vi "main_ui.vi"() -> ()   [LabVIEW 2018]
uses:
  <vilib>/Utility/miscctls.llb/LVPointDoubleTypeDef.ctl
  <vilib>/Analysis/1siggen.llb/Ramp Pattern by Samples.vi
  src/GLOBAL_VAR.vi
  <vilib>/Analysis/NI_AALBase.lvlib
panel:
  in  "T2_open":bool caption="Open T1"
  in  "parameters_z-scan":T1={"dwell_time_ms"=10.0, "q_steps"=20, "span_um"=2.0, "refocus"=TRUE}
  in  "parameters_xy-scan":T2={"image_size_xy_um"=0.5, "frame_size_xy_px"=20, "dwell_time_ms"=1.0}
  in  "continious_recenter":bool
  in  "recenter":bool caption="Laser"
  out "Laser power [mW]":dbl caption="Power" format="%.3f"
  in  "laser_on-off":bool caption="Laser"
  in  "T1_open":bool caption="Open T1"
  in  "esr_start":bool caption="Open ESR"
  in  "stop":bool
  in  "scan_start":bool
  in  "live-scan":bool
  out "ESR_stack":dbl[][](graph)
  out "X":dbl caption="X Rel" format="%.3f"
  out "Y":dbl caption="Y Rel" format="%.3f"
  out "XY Graph 2":cluster{"Value":dbl[], "Ramp Pattern":dbl[]}(graph)={"Value"=[-75.0, -71.93877551020408, -68.87755102040816, -65.81632653061224, -62.755102040816325, -59.69387755102041, -56.63265306122449, -53.57142857142857, -50.51020408163265, -47.44897959183673, -44.38775510204081, -41.3265306122449, -38.26530612244898, -35.204081632653065, -32.142857142857146, -29.081632653061227, -26.02040816326531, -22.95918367346939, -19.89795918367347, -16.836734693877553, -13.775510204081634, -10.714285714285722, -7.653061224489804, -4.591836734693885, -1.5306122448979664, 1.5306122448979522, 4.591836734693871, 7.6530612244897895, 10.714285714285708, 13.775510204081627, 16.836734693877546, 19.897959183673464, 22.959183673469383, 26.0204081632653, 29.08163265306122, 32.14285714285714, 35.20408163265306, 38.265306122448976, 41.326530612244895, 44.38775510204081, 47.44897959183673, 50.51020408163265, 53.571428571428555, 56.63265306122449, 59.69387755102039, 62.755102040816325, 65.81632653061223, 68.87755102040816, 71.93877551020407, 75.0], "Ramp Pattern"=[0.0, 0.0, 0.0, 0.0, 0.0, 0.0, 0.0, 0.0, 0.0, 0.0, 0.0, 0.0, 0.0, 0.0, 0.0, 0.0, 0.0, 0.0, 0.0, 0.0, 0.0, 0.0, 0.0, 0.0, 0.0, 0.0, 0.0, 0.0, 0.0, 0.0, 0.0, 0.0, 0.0, 0.0, 0.0, 0.0, 0.0, 0.0, 0.0, 0.0, 0.0, 0.0, 0.0, 0.0, 0.0, 0.0, 0.0, 0.0, 0.0, 0.0]}
  out "XY Graph":cluster{"Value":dbl[], "Ramp Pattern":dbl[]}(graph)={"Value"=[0.0, 0.0, 0.0, 0.0, 0.0, 0.0, 0.0, 0.0, 0.0, 0.0, 0.0, 0.0, 0.0, 0.0, 0.0, 0.0, 0.0, 0.0, 0.0, 0.0, 0.0, 0.0, 0.0, 0.0, 0.0, 0.0, 0.0, 0.0, 0.0, 0.0, 0.0, 0.0, 0.0, 0.0, 0.0, 0.0, 0.0, 0.0, 0.0, 0.0, 0.0, 0.0, 0.0, 0.0, 0.0, 0.0, 0.0, 0.0, 0.0, 0.0], "Ramp Pattern"=[-75.0, -71.93877551020408, -68.87755102040816, -65.81632653061224, -62.755102040816325, -59.69387755102041, -56.63265306122449, -53.57142857142857, -50.51020408163265, -47.44897959183673, -44.38775510204081, -41.3265306122449, -38.26530612244898, -35.204081632653065, -32.142857142857146, -29.081632653061227, -26.02040816326531, -22.95918367346939, -19.89795918367347, -16.836734693877553, -13.775510204081634, -10.714285714285722, -7.653061224489804, -4.591836734693885, -1.5306122448979664, 1.5306122448979522, 4.591836734693871, 7.6530612244897895, 10.714285714285708, 13.775510204081627, 16.836734693877546, 19.897959183673464, 22.959183673469383, 26.0204081632653, 29.08163265306122, 32.14285714285714, 35.20408163265306, 38.265306122448976, 41.326530612244895, 44.38775510204081, 47.44897959183673, 50.51020408163265, 53.571428571428555, 56.63265306122449, 59.69387755102039, 62.755102040816325, 65.81632653061223, 68.87755102040816, 71.93877551020407, 75.0]}
  out "scan_image":dbl[][](graph)
  out "wavechart_01":dbl(graph)
  in  "Tab Control":T3(tab)
  in  "counting_start":bool
  out "counts":dbl format="%.3e"
  in  "counts_dwell_time":dbl=30.0 caption="Dwell time [ms] :" min=0.0
  in  "pos-zero":bool caption="Blank Button"
  in  "scan_direction":enum32{"0", "1"}(radio)=enum."1" caption="Scan direction:"
  in  "frame_size_x_px":i32=100 caption="image_size_x"
  out "frame_size_y_px":i32=100 caption="image_size_y"
  out "pixel_size_z_um":dbl format="%#_3g"
  out "pixel_size_x_um":dbl=1.5 format="%#_3g"
  out "pixel_size_y_um":dbl=1.5 format="%#_3g"
  in  "pixel_dwell_ms":dbl=1.0 caption="Dwell time:"
  out "time_frame_s":dbl=10.0 caption="Time per frame:"
  in  "cursor-reset":bool caption="Blank Button"
  in  "pos-start_y":dbl caption="Y:" format="%#.3g"
  in  "pos-start_x":dbl caption="X:" format="%#.3f"
  in  "pos-start_cursor":bool caption="Blank Button"
  in  "pos_start":enum32{"bottom-left", "center"}(radio)=enum."center"
  in  "image_size_x_um":dbl=150.0 caption="X:"
  out "image_size_y_um":dbl=150.0 caption="Y:"
  in  "pos_z":dbl(slide) caption="Z:" scale=0.0..200.0
  in  "focus_z":dbl caption="Focus :" min=0.0 max=200.0 step=0.001 format="%.3f"
  in  "focus_dwell_ms":dbl=100.0 caption="Dwell :"
  in  "focus_q_steps":i32=100 caption="Steps :"
  in  "focus_z_end":dbl=100.0 caption="End :"
  in  "focus_z_start":dbl caption="Start :"
  in  "focus_start":bool
  out "timeseries-rem_time":string caption="Remaining time :"
  in  "timeseries-autofocus":enum16{"No autofocus", "Max x-y", "Center"}(ring) caption="Autofocus :"
  out "timeseries-current_image":dbl caption="Current scan :" format="%#.3f"
  out "timeseries-total_images":dbl=1.0 caption="Total scans :" format="%#.3f"
  in  "timeseries-start":bool
  in  "timeseries-period":dbl caption="Period :" format="%#.3f"
  in  "timeseries-stopdate":timestamp=timestamp(3557915984.536238 s since 1904-01-01) caption="Stop at :" format="%<%X\n%x>T"
  out "timeseries-next_scan":timestamp caption="Next scan at :" format="%<%X\n%x>T"
  in  "Z-stack_enable":bool
  in  "z-stack_slices":i32=1 caption="Slices :" min=1 step=1
  out "z-stack_step_size":dbl caption="Step size :" format="%#.4f"
  in  "Z-stack_tabs":enum32{"From-To", "Centering"}(tab)
  in  "z-stack-set_to":bool
  in  "z-stack-set_from":bool
  in  "z-stack_to":dbl=100.0 caption="To :"
  in  "z-stack_from":dbl caption="From :"
  in  "z-stack-set_center":bool
  in  "z-stack_size":dbl=10.0 caption="Size :"
  in  "z-stack_center":dbl=5.0 caption="Center :"
  in  "z-stack_pos":i32(slide)=1 caption="Z slice :" min=1 step=1 scale=1.0..1.1
  in  "current_z":dbl caption="Z :" min=0.0 max=100.0 step=0.0001 format="%.4f"
  in  "current_y":dbl caption="Y :" min=-10.0 max=10.0 step=0.0001 format="%.4f"
  in  "current_x":dbl caption="X :" min=-10.0 max=10.0 step=0.0001 format="%.4f"
  in  "XY Max focus?":bool
  in  "X Zero":dbl format="%.3f"
  in  "Y Zero":dbl format="%.3f"
  in  "X Rel":dbl format="%.3f"
  in  "Y Rel":dbl format="%.3f"
  out "upos-xy_control":cluster{"X":dbl, "Y":dbl}[](graph)
  in  "upos-stop":bool
  in  "upos-x":dbl caption="X:" min=0.0 max=7.0 format="%.3f"
  in  "upos-y":dbl caption="Y:" min=0.0 max=7.0 format="%.3f"
  out "upos-cpos_y":dbl format="%#.3f"
  out "upos-cpos_x":dbl format="%#.3f"
  out "upos-state_x":u32 caption="X:"
  out "upos-state_y":u32 caption="Y:"
  in  "tiles-overlap":dbl=10.0 caption="Overlap :"
  out "tile_progress":u8(slide) caption="Progress :" scale=0.0..100.0
  out "tile_remaining_tiles":dbl caption="Remaining\ntiles :"
  out "tile_remaining_time":dbl caption="Remaining\ntime :"
  in  "tile-scan_start":bool
  in  "tile_tiles-size":enum32{"tiles", "size"}(radio)=enum."size"
  out "tile_q-tiles_y":dbl=1.0 caption="Y :"
  in  "tile_q-tiles_x":dbl=1.0 caption="X :"
  out "tile_size_y_um":dbl=10.0 caption="Y:"
  in  "tile_size_x_um":dbl=10.0 caption="Size :"
  in  "tile_start_y_mm":dbl caption="Y:" format="%#.3g"
  in  "tile_start_x_mm":dbl caption="X:" format="%#.3f"
  out "esr_generator_ok":bool caption="Generator\nstatus :"
  out "esr_current_run":i32 caption="Run :"
  in  "esr_out_enable":bool caption="Output on/off :"
  out "esr_power_led":bool
  out "esr_remain":i32 caption="Remain :"
  in  "esr_repetitions":i32=1 caption="Repetitions" min=1 max=1000 step=1
  in  "esr_dwell_time":ext=0.09999999974525053 caption="Dwell Time :" format="%.3f"
  in  "esr_step_size":ext=2500000.0 caption="Step size :" format="%.2p"
  in  "esr_freq_stop":ext=3000000000.0 caption="Freq Stop :" format="%.2p"
  in  "esr_freq_start":ext=2800000000.0 caption="Freq Start :" format="%.2p"
  out "esr_total_time":ext=8120.249980327117 caption="Total time :"
  in  "esr_power":ext=5.999999061226845 caption="Power :" format="%.2f"
  in  "live_scan_direction":enum32{"0", "1"}(radio)=enum."1" caption="Scan direction:"
  in  "live_frame_size_x_px":i32=50 caption="image_size_x"
  in  "live_pixel_dwell_ms":dbl=0.5 caption="Dwell time:"
  in  "objective":u16(ring)=1 items=["Raw scale (volts)", "UPlanSApo 100x / 1,40 Oil", "UPlanSApo 40X / 0,95 Air"]
  in  "file_save":bool
  in  "file_autosave":bool
  in  "file_path":path caption="Folder :"
  in  "file_name":string caption="Name :"
  in  "save_tiff":bool
  in  "save_txt":bool
  # "Relative cursor position [um]"
  # "Scanning area [mm]"
  # "Size:"
  # "x"
  # "Position:"
  # "Acquisition"
  # "Frame size:"
  # "x"
  # "px"
  # "ms"
  # "Pixel size [mm] :"
  # "x"
  # "x"
  # "Seconds"
  # "Manual focus [mm]"
  # "Auto-focus [mm]"
  # "ms"
  # "Photon counting"
  # "Time series"
  # "[s]"
  # "Z stack [mm]"
  # "Set position [mm]"
  # "Positioners (xy motors)"
  # "Absolute"
  # "Zeros"
  # "Relative"
  # "Status"
  # "State :"
  # "Position :"
  # "Tiles scan"
  # "Start position [mm]:"
  # "mm"
  # "mm"
  # "mm"
  # "min"
  # "Sweep"
  # "Hz"
  # "Hz"
  # "Hz"
  # "ms"
  # "dBm"
  # "s"
  # "Objective"
  # "Live scan"
  # "Frame size:"
  # "px"
  # "ms"
  # "Save"
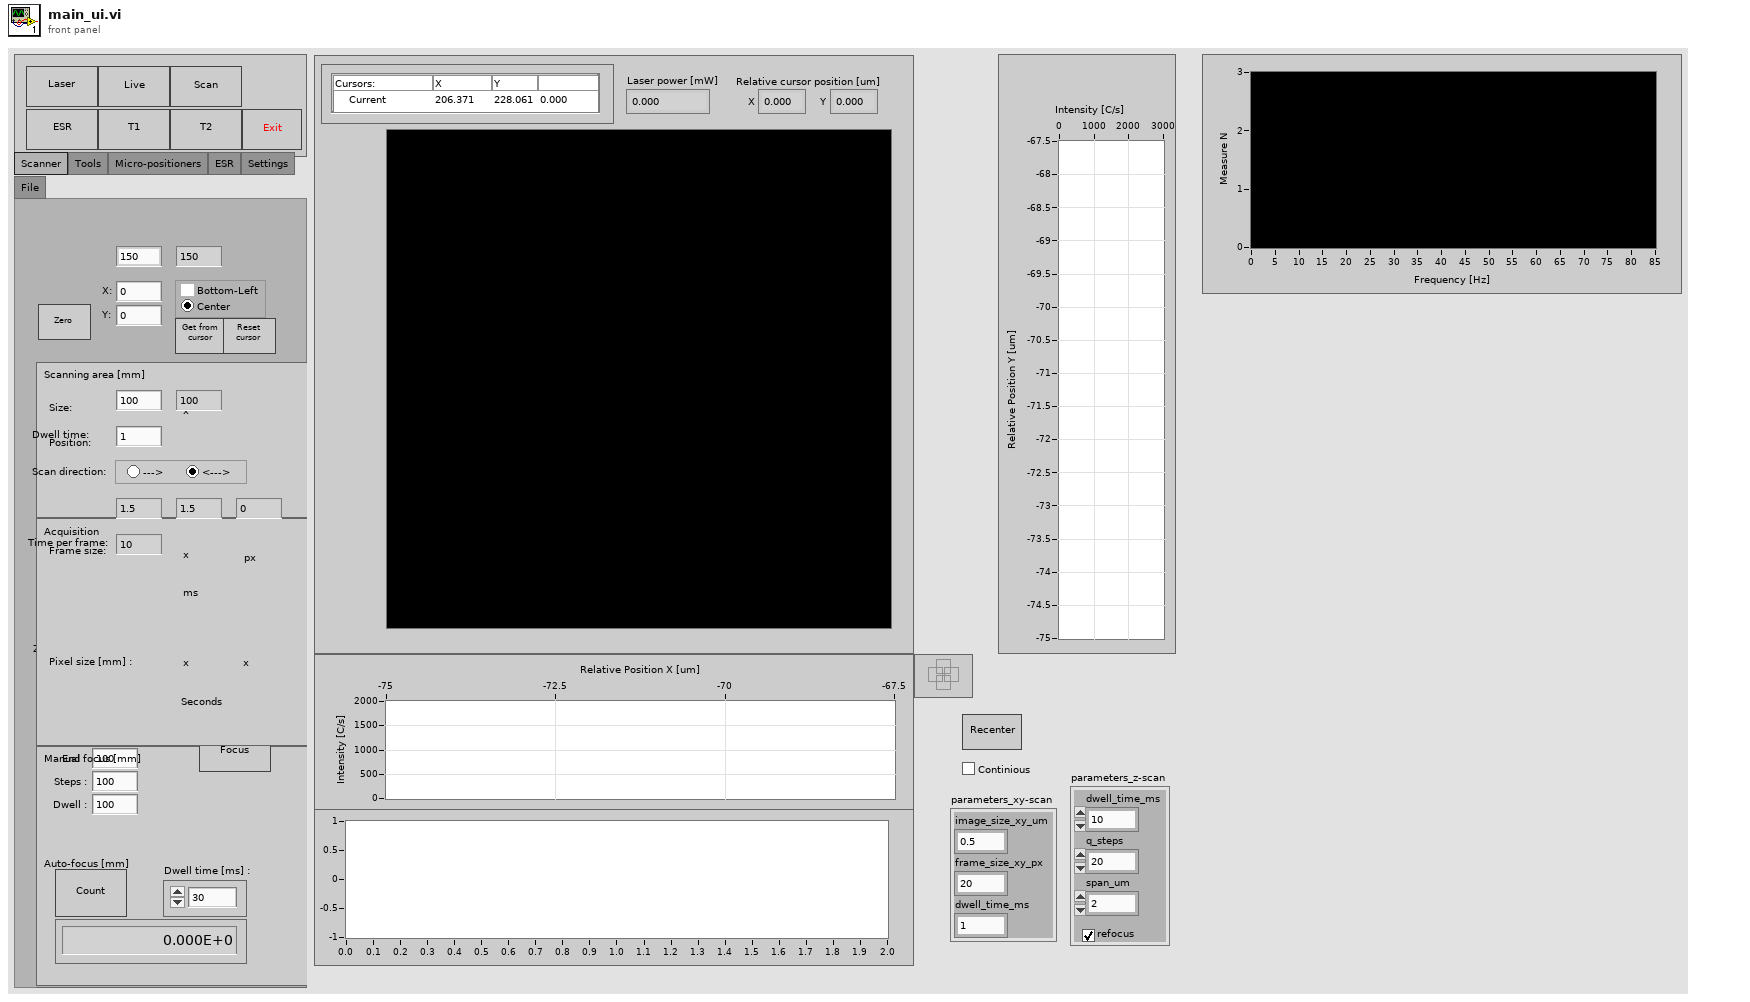
[diagram p1: front panel]
types:
  T1 = cluster{"dwell_time_ms":dbl, "q_steps":u32, "span_um":dbl, "refocus":bool}
  T2 = cluster{"image_size_xy_um":dbl, "frame_size_xy_px":u32, "dwell_time_ms":dbl}
  T3 = enum32{"Scanner", "Tools", "Micro-positioners", "ESR", "Settings", "File"}
  T4 = cluster{"status_x":dbl, "status_y":dbl, "status_z":dbl, "pos_x":dbl, "pos_y":dbl, "pos_z":dbl}
  T5 = cluster{enum16{"standby", "domove", "dostop", "exit", "status"}, dbl, dbl, dbl}
  T6 = typedef "LVPointDoubleTypeDef.ctl" = cluster{"X":dbl, "Y":dbl}
  T7 = enum8{"Enabled", "Disabled", "Disabled and Grayed Out"}
  T8 = cluster{"overlap":dbl, "pos-xy_start":cluster{"pos-x_start":dbl, "pos-y_start":dbl}, "pos-xy_end":cluster{"pos-x_end":dbl, "pos-y_end":dbl}, "pos-xy_ref":cluster{"pos-x_start":dbl, "pos-y_start":dbl}}
  T9 = cluster{"z_start":dbl, "z_end":dbl, "q_steps":i32, "dwell_time_ms":dbl}
  T10 = cluster{"image_size":dbl, "image_xy_start":cluster{"image-x_start":dbl, "image-y_start":dbl}, "pixel_dwell_ms":dbl, "frame_size_x_px":i32, "scan_direction":enum32{"0", "1"}, "pos_start":enum32{"bottom-left", "center"}}
  T11 = cluster{"nano-position_X_um":sgl, "nano-position_Y_um":sgl, "nano-position Z_um":sgl}
  T12 = enum16{"Standby", "doScan", "doCount", "doFocus", "doLiveScan", "do3DScan"}
  T13 = enum16{"Standby", "doScan", "doCount", "doFocus", "doLiveScan"}
  T14 = enum16{"Standby", "doScan", "doCount", "doFocus", "doLiveScan", "do3DScan", "changeZslice", "doESR", "doTileScan", "doStartPos", "doTimeseries"}
  T15 = enum16{"Standby", "doScan", "doCount", "doFocus"}
  T16 = enum16{"Standby", "doScan", "doCount", "doFocus", "doLiveScan", "do3DScan", "changeZslice", "doESR", "doTileScan", "doStartPos", "doTimeseries", "saveImage", "doT1", "doRecenter"}
  T17 = enum16{"Standby", "doScan", "doCount", "doFocus", "doLiveScan", "do3DScan", "changeZslice"}
  T18 = enum16{"Standby", "doScan", "doCount", "doFocus", "doLiveScan", "do3DScan", "changeZslice", "doESR"}
  T19 = enum16{"Standby", "doScan", "doCount", "doFocus", "doLiveScan", "do3DScan", "changeZslice", "doESR", "doTileScan"}
  T20 = enum16{"standby", "domove", "dostop", "exit", "status"}
  T21 = enum16{"Standby", "doScan", "doCount", "doFocus", "doLiveScan", "do3DScan", "changeZslice", "doESR", "doTileScan", "doStartPos", "doTimeseries", "saveImage", "doT1"}
  T22 = enum16{"Standby", "doScan", "doCount", "doFocus", "doLiveScan", "do3DScan", "changeZslice", "doESR", "doTileScan", "doStartPos", "doTimeseries", "saveImage", "doT1", "doRecenter", "doT2"}
  T23 = enum16{"Standby", "doScan", "doCount", "doFocus", "doLiveScan", "do3DScan", "changeZslice", "doESR", "doTileScan", "doStartPos", "doTimeseries", "saveImage"}
  T24 = cluster{enum16{"standby", "domove", "dostop", "exit", "status"}, "Value":dbl, "Value":dbl, "Value":dbl}
  T25 = cluster{enum16{"standby", "domove", "dostop", "exit", "status"}, dbl, dbl, "Value":dbl}
  T26 = cluster{enum16{"standby", "domove", "dostop"}, "X":dbl, "Y":dbl, dbl}
  T27 = cluster{enum16{"standby", "domove", "dostop", "exit"}, "upos-x":dbl, "upos-y":dbl, dbl}
  T28 = cluster{enum16{"standby", "domove", "dostop", "exit"}, dbl, dbl, dbl}
  T29 = cluster{"pos-start_x":dbl, "pos-start_y":dbl, "focus_z":dbl}
  T30 = cluster{"file_path":path, "file_name":string, "image":dbl[][][], "image_size_xy":cluster{"image_size_x_um":sgl, "image_size_y_um":sgl}, "pixel_dwell_time_ms":sgl, "Laser_power_mW":sgl, "pixel_size":dbl, "tile_ij":cluster{"tile_i":i32, "tile_j":i32}, "Objective":string, "ColorMarkers":cluster{dbl, u32}[], "timestamp":timestamp, "micro-position-xyz":cluster{"micro-position_x_mm":sgl, "micro-position_y_mm":sgl, "micro-position_z_mm":sgl}, "zero_xyz":cluster{"zero_x_mm":dbl, "zero_y_mm":dbl, "zero_z_mm":dbl}, "nano-position-xyz":cluster{"nano-position_x_V":sgl, "nano-position_y_V":sgl, "nano-position_z_V":sgl}, "Kxyz":cluster{"Kx_V/um":sgl, "Ky_V/um":sgl, "Kz_V/um":sgl}}
  T31 = cluster{"image_size_x_um":dbl, "image_size_x_um":dbl}
  T32 = cluster{"esr_repetitions":i32, "esr_power":ext, "esr_freq_start":ext, "esr_freq_stop":ext, "esr_step_size":ext, "esr_dwell_time":ext}
  T33 = cluster{"Cursor.Cursor X":dbl, "Cursor.Cursor Y":dbl, "focus_z":dbl}
  T34 = cluster{"tile_start_x_mm":dbl, "tile_start_y_mm":dbl}
  T35 = cluster{"Value":dbl, "Value":dbl, "Value":i32, "Value":bool}
  T36 = cluster{"timeseries-current_image":refnum<vi>, "scan_image":refnum<vi>, "timeseries-start":refnum<vi>, "timeseries-next_scan":refnum<vi>, "timeseries-rem_time":refnum<vi>}
  T37 = cluster{"X Zero":dbl, "Y Zero":dbl, "upos-y":dbl}
  T38 = cluster{"Cursor.Cursor X":dbl, "Cursor.Cursor Y":dbl, "Value":dbl}
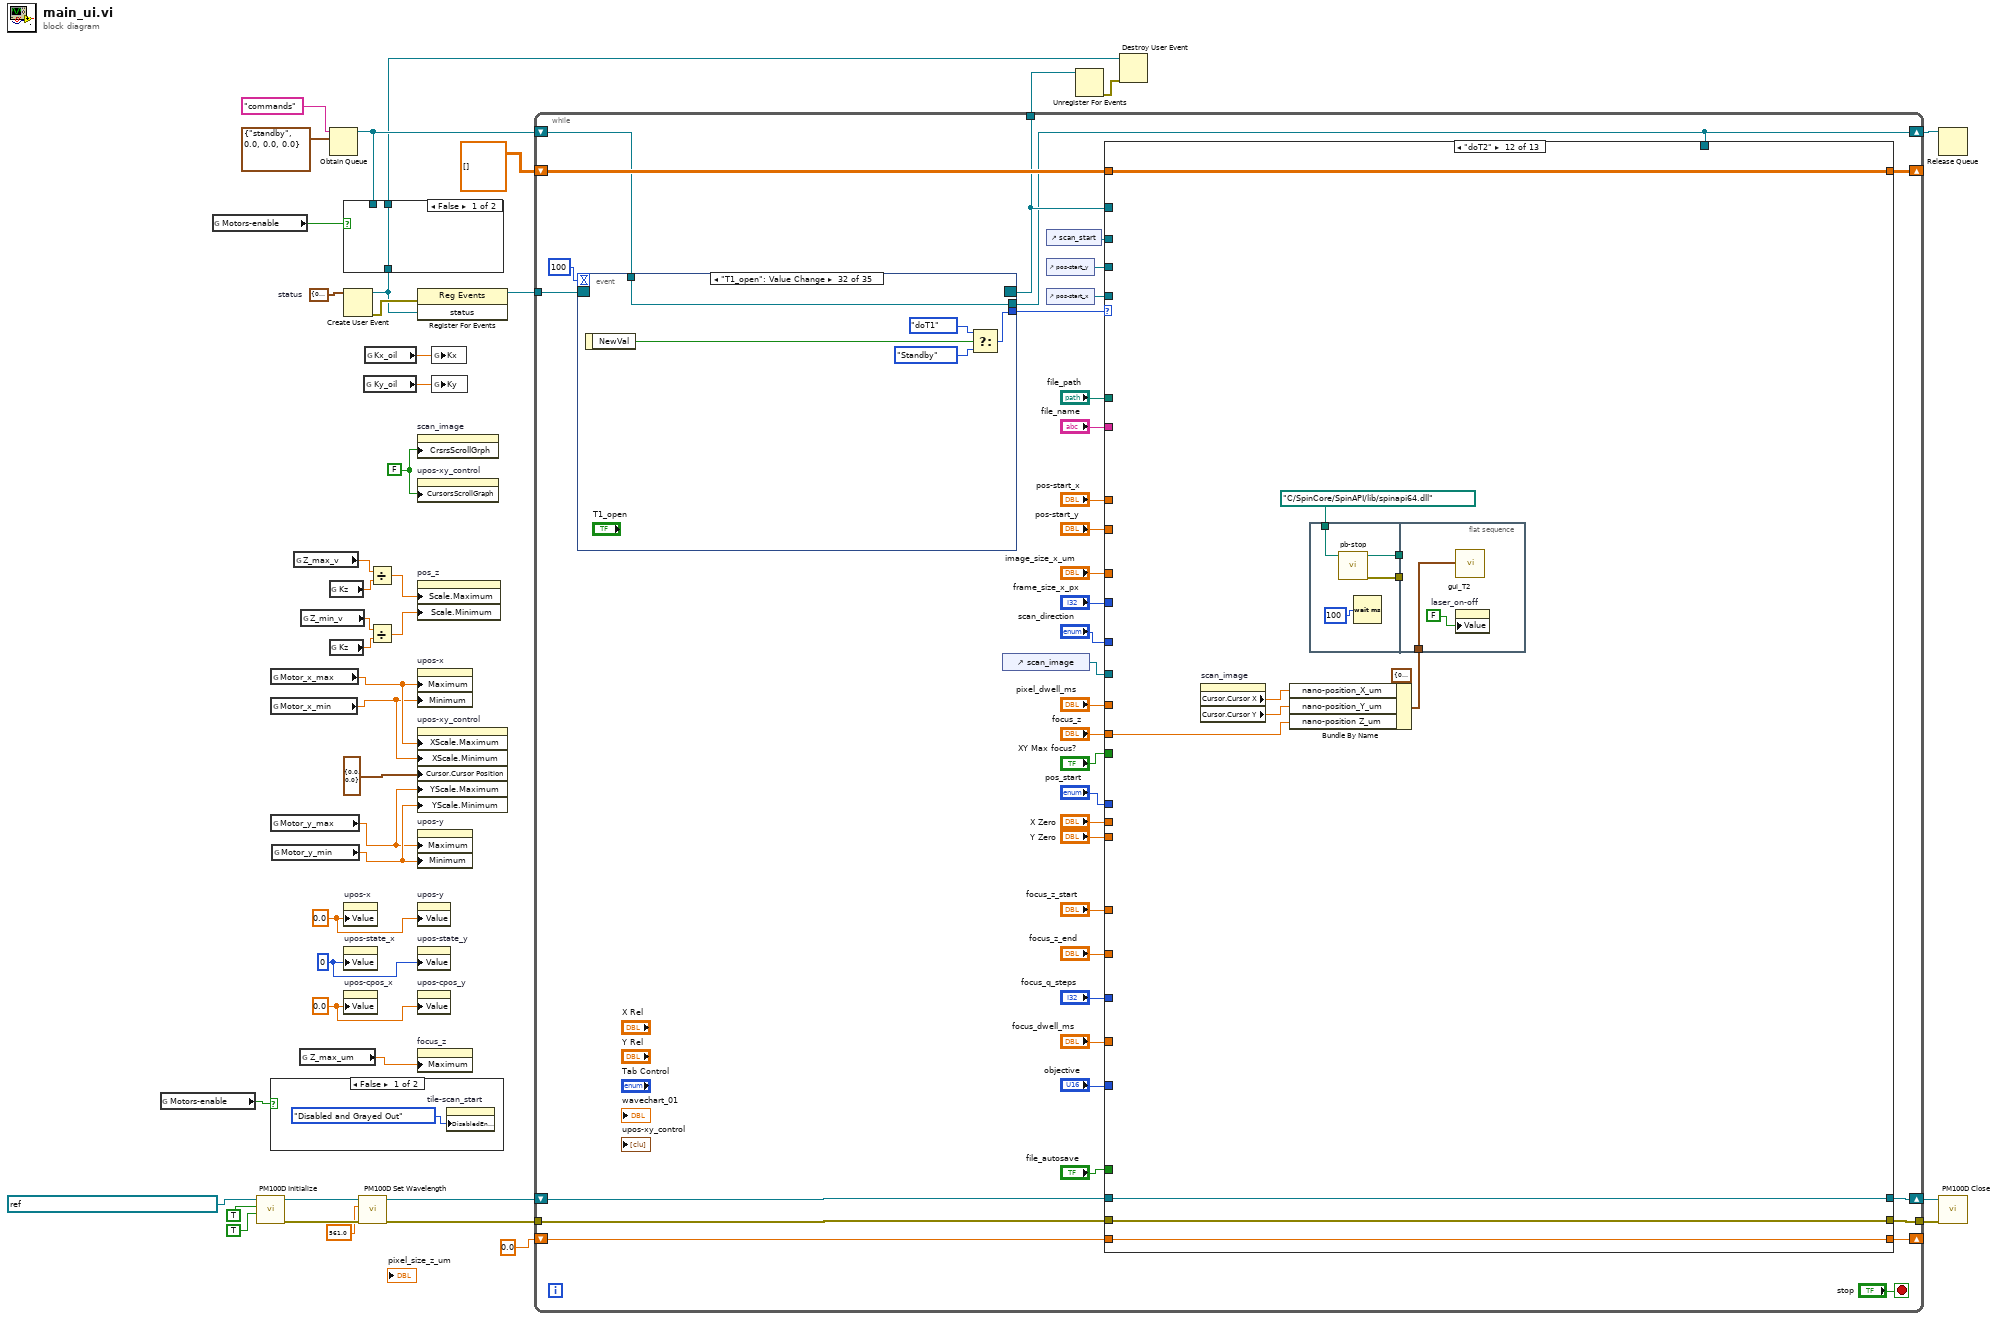
[diagram p0: block diagram]
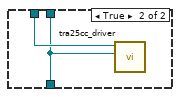
[diagram p2: hidden frame]
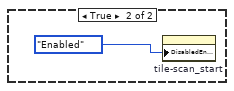
[diagram p3: hidden frame]
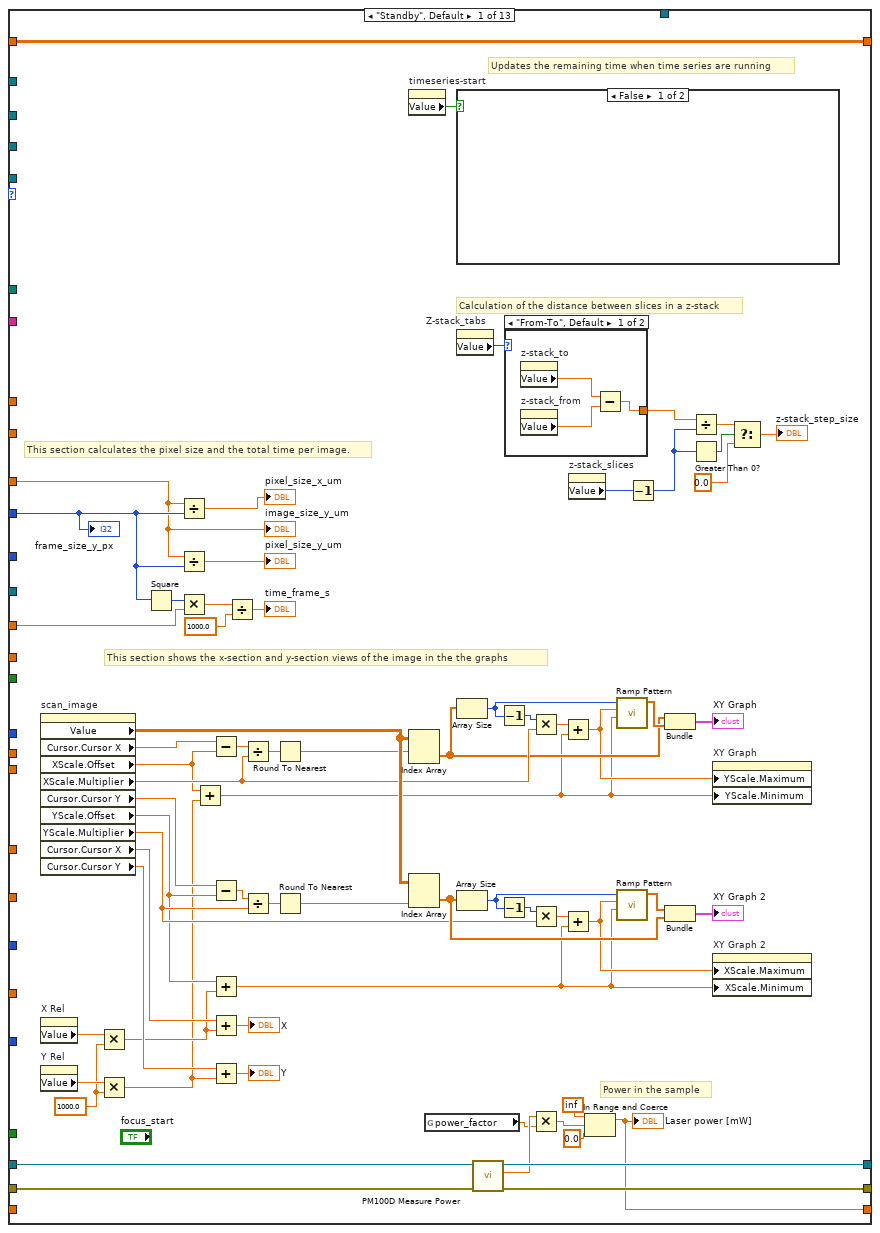
[diagram p4: hidden frame]
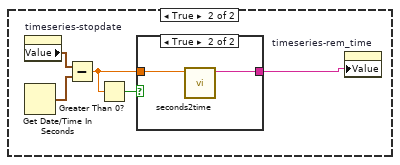
[diagram p5: hidden frame]
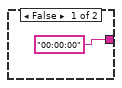
[diagram p6: hidden frame]
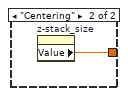
[diagram p7: hidden frame]
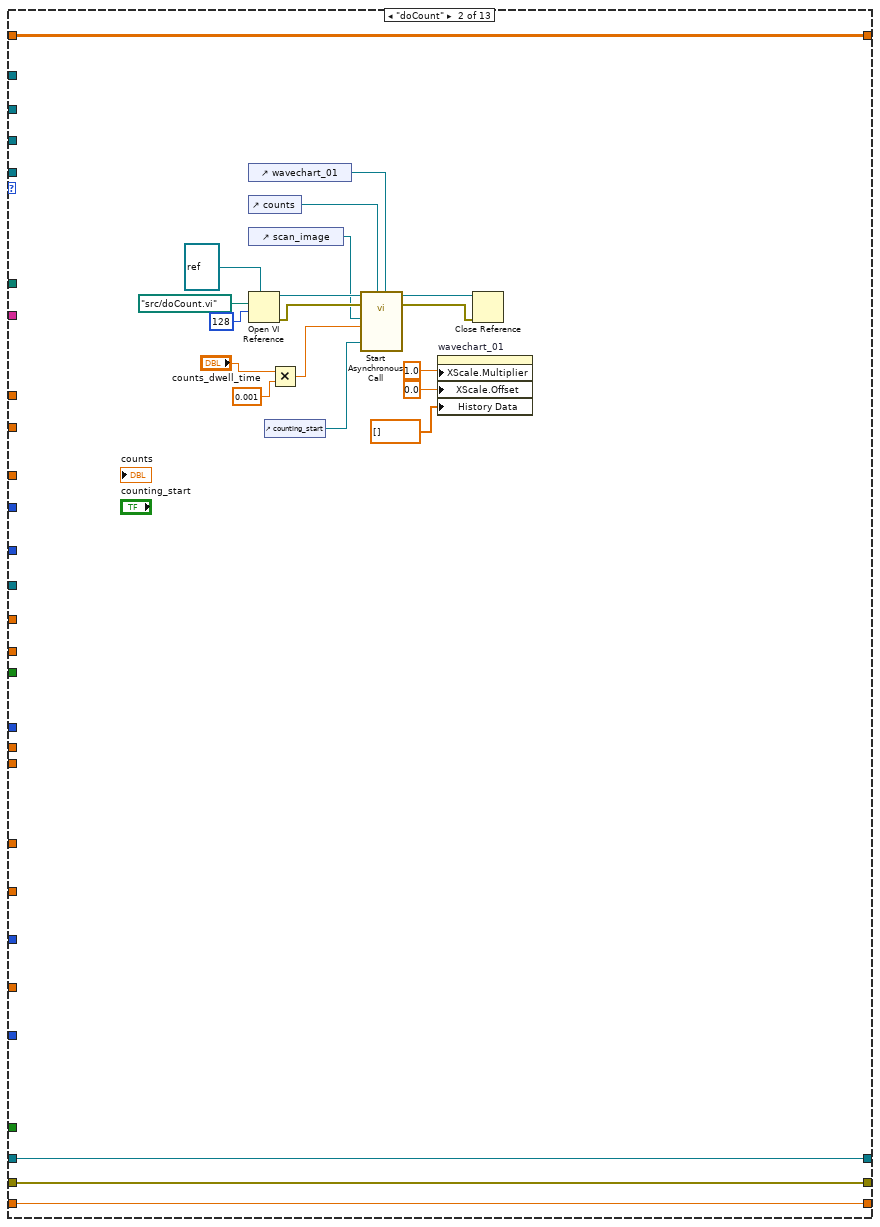
[diagram p8: hidden frame]
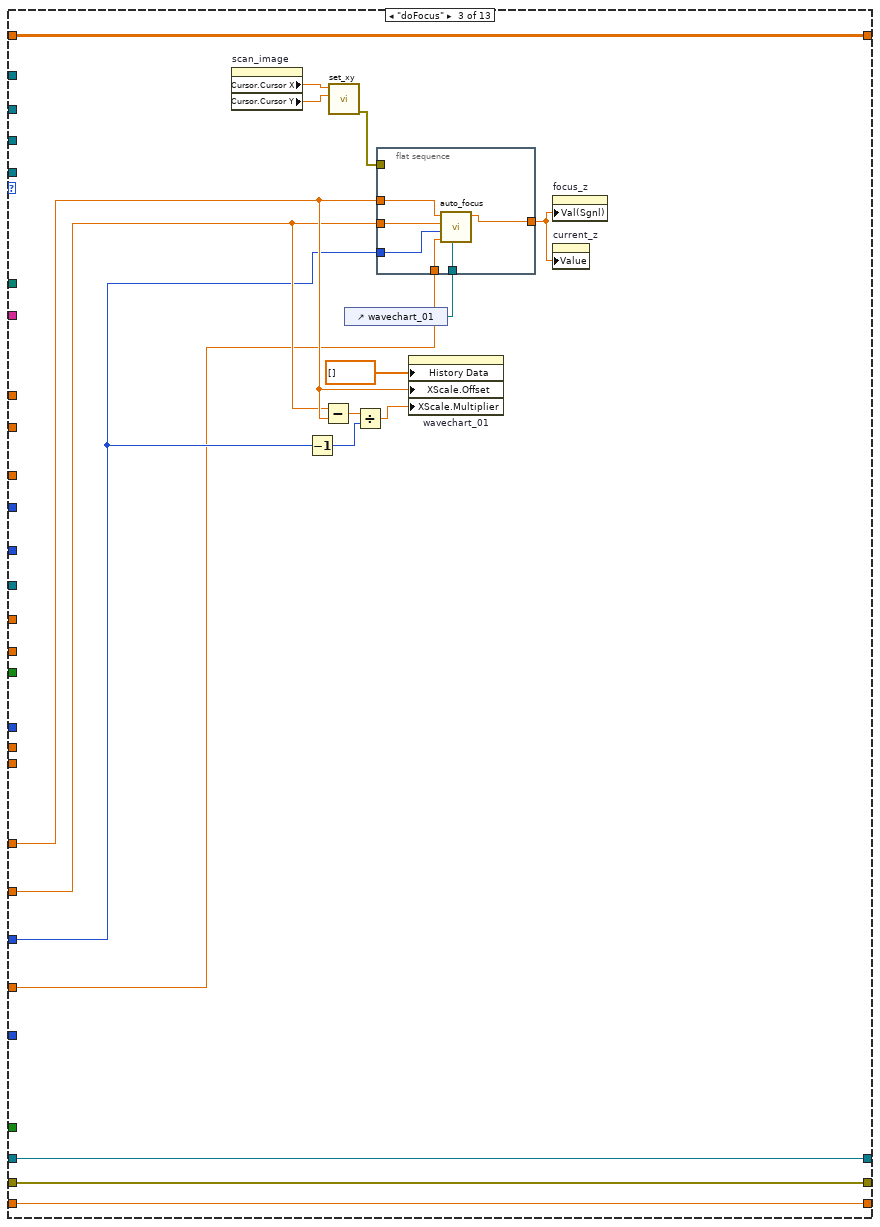
[diagram p9: hidden frame]
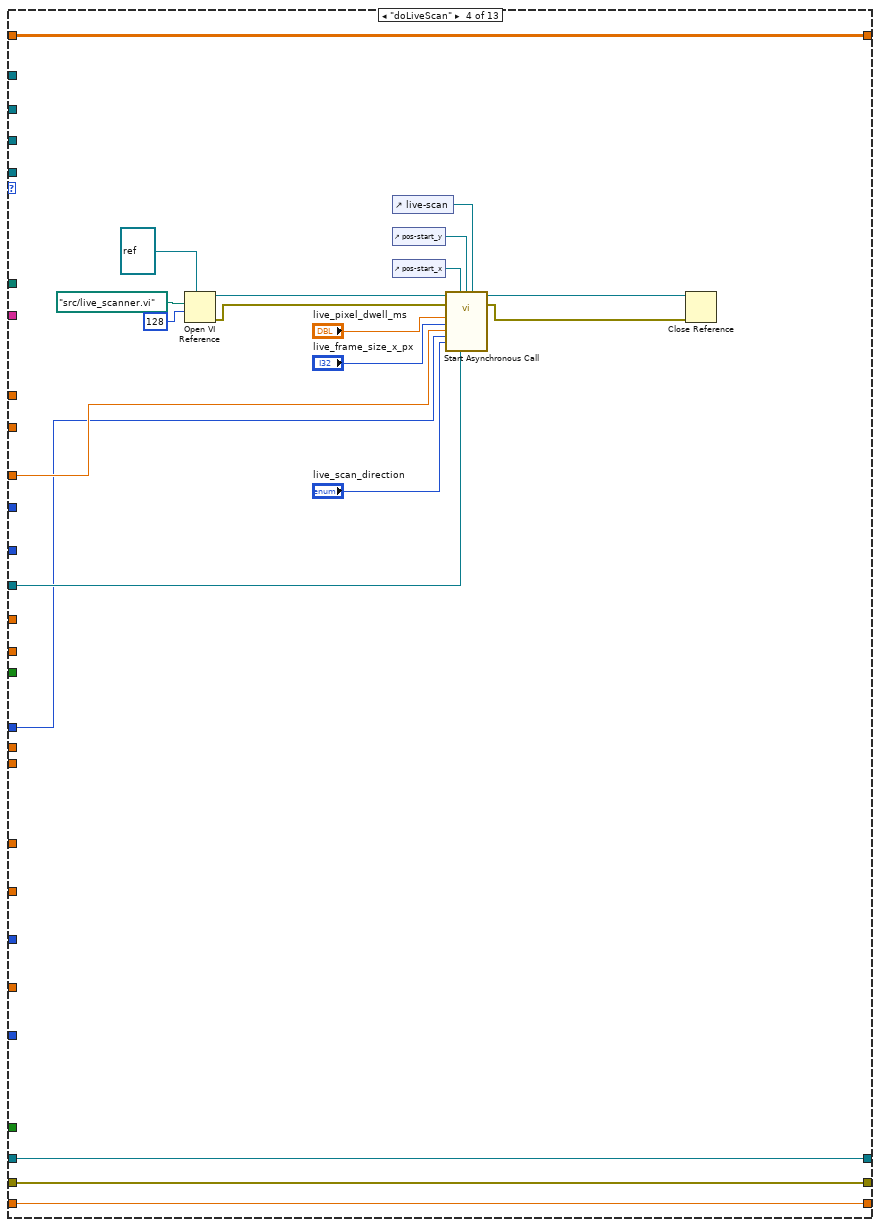
[diagram p10: hidden frame]
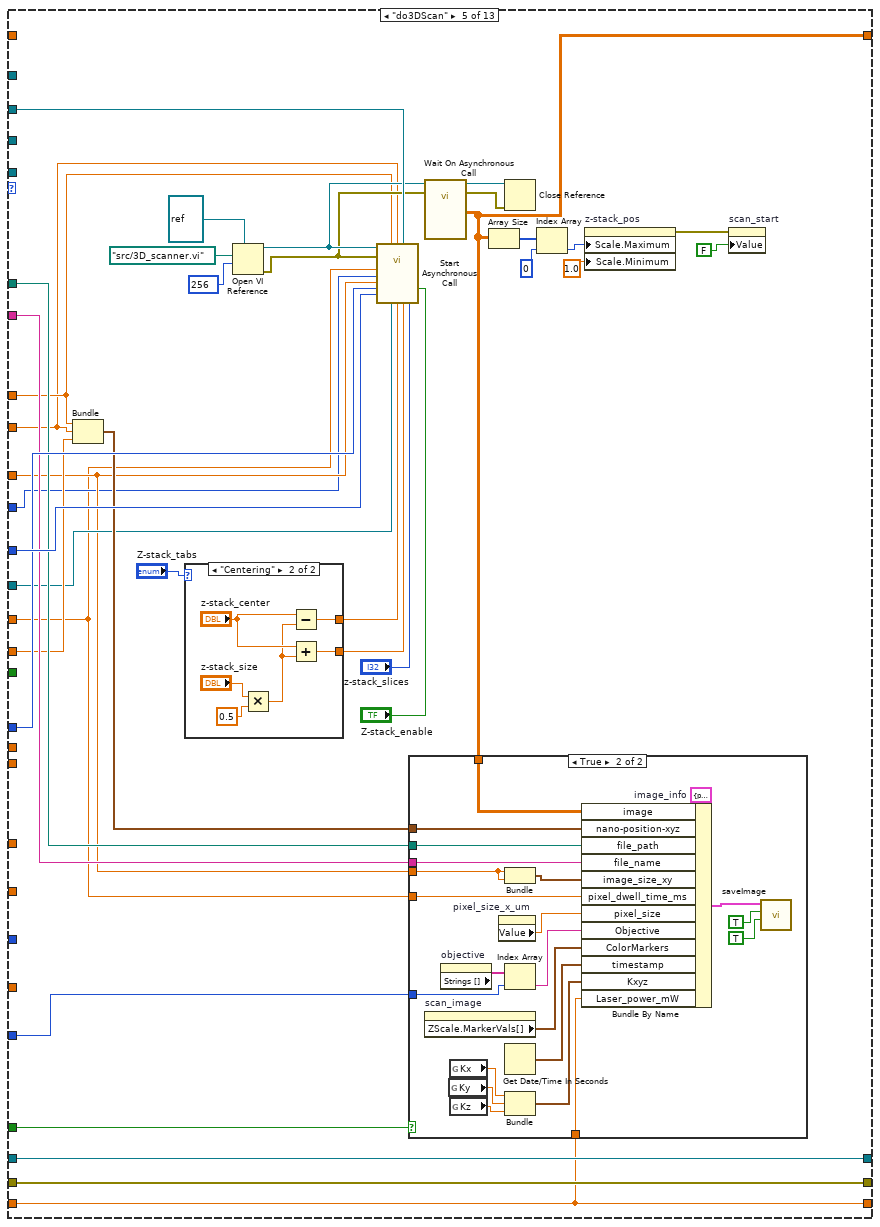
[diagram p11: hidden frame]
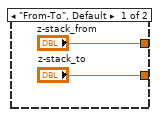
[diagram p13: hidden frame]
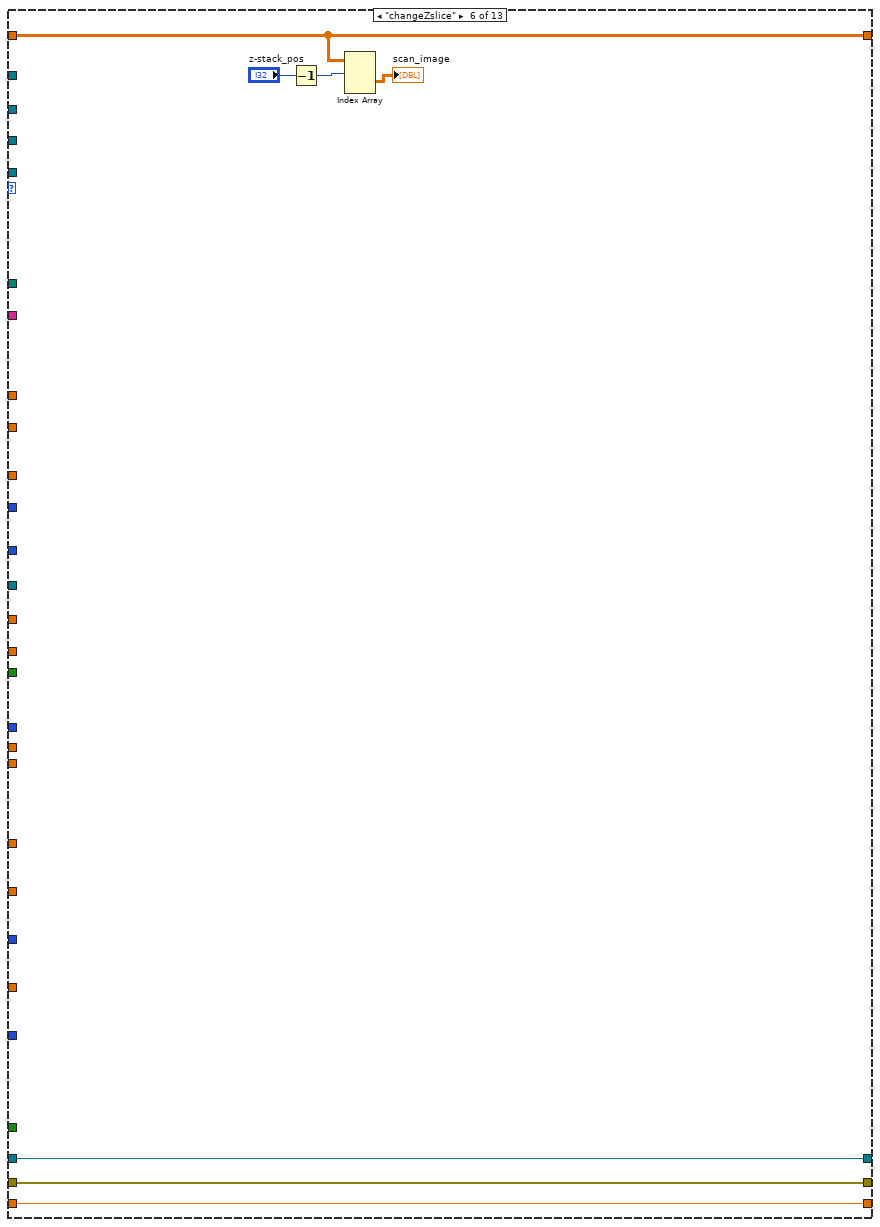
[diagram p14: hidden frame]
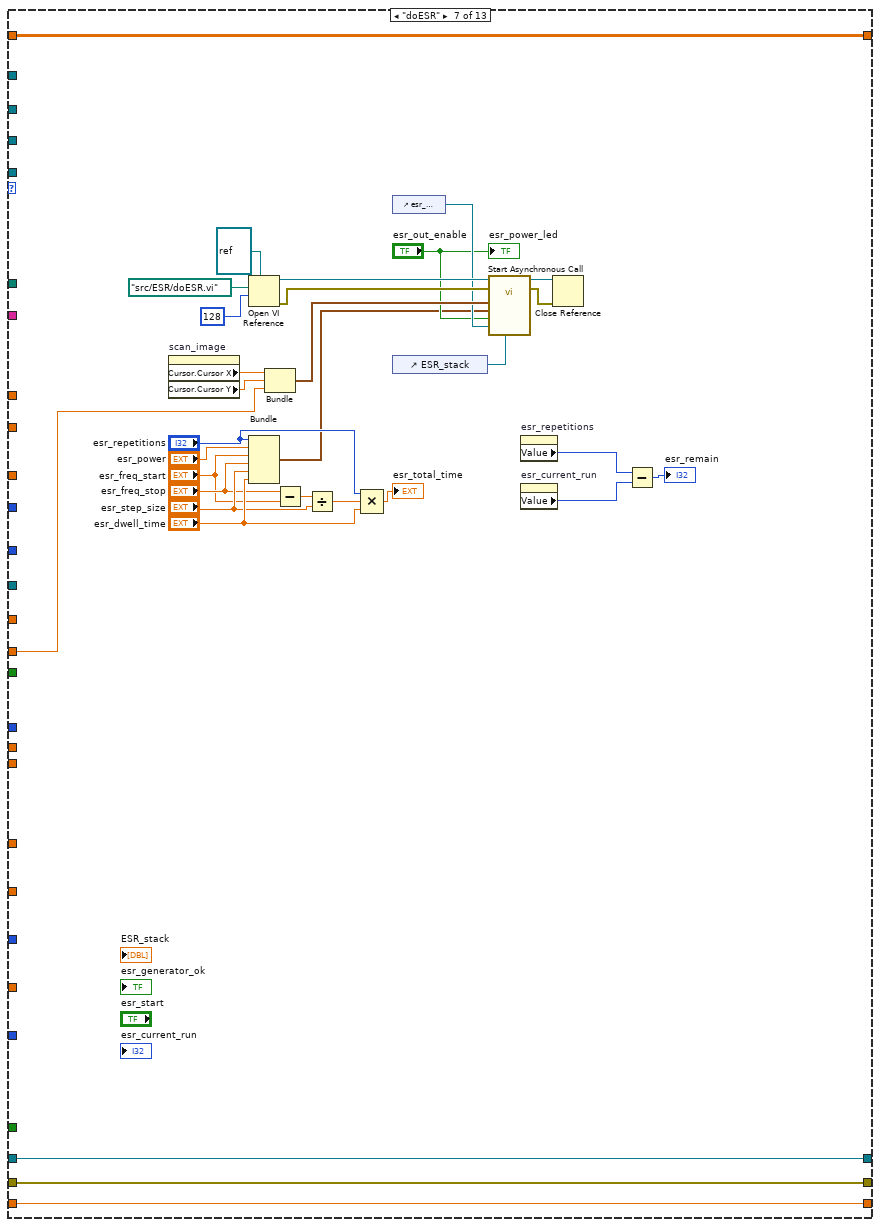
[diagram p15: hidden frame]
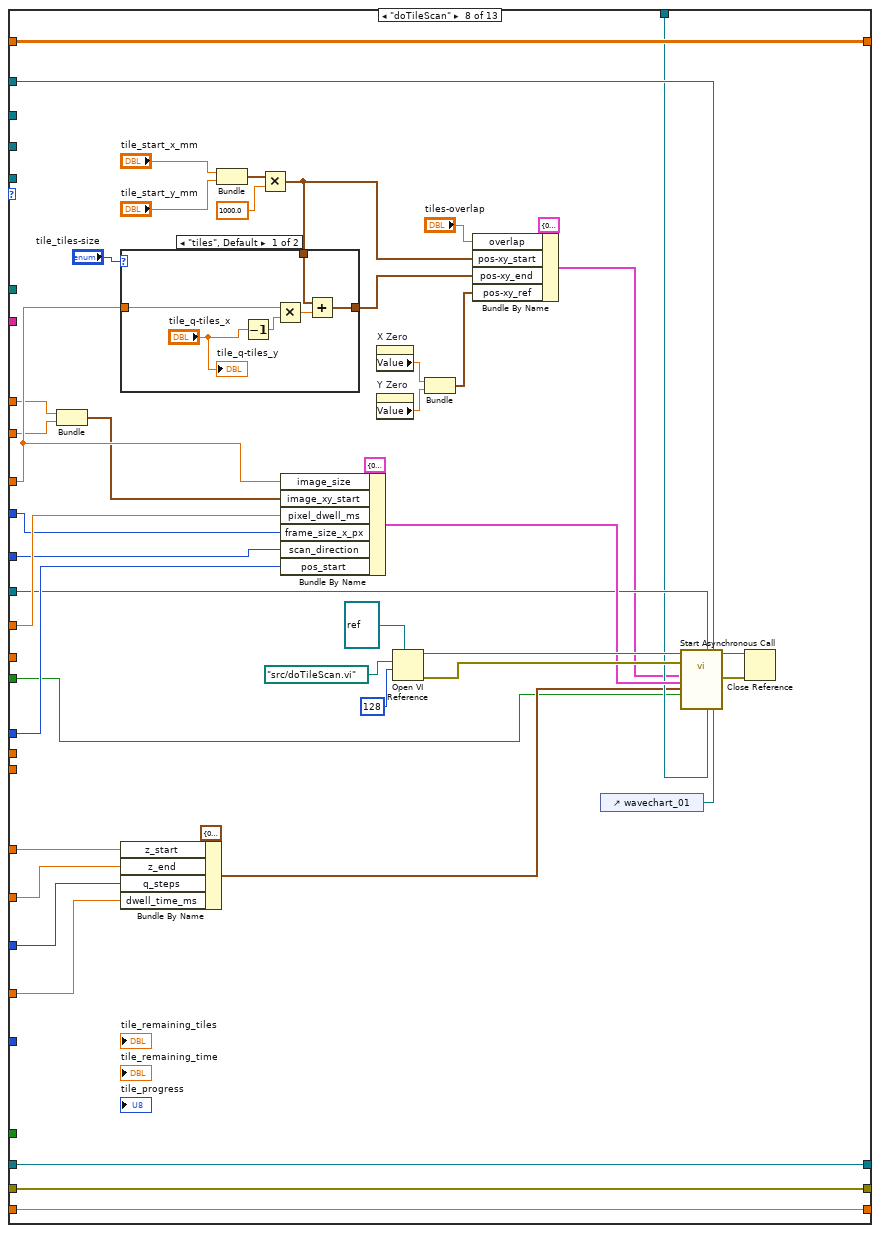
[diagram p16: hidden frame]
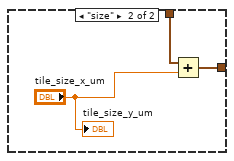
[diagram p17: hidden frame]
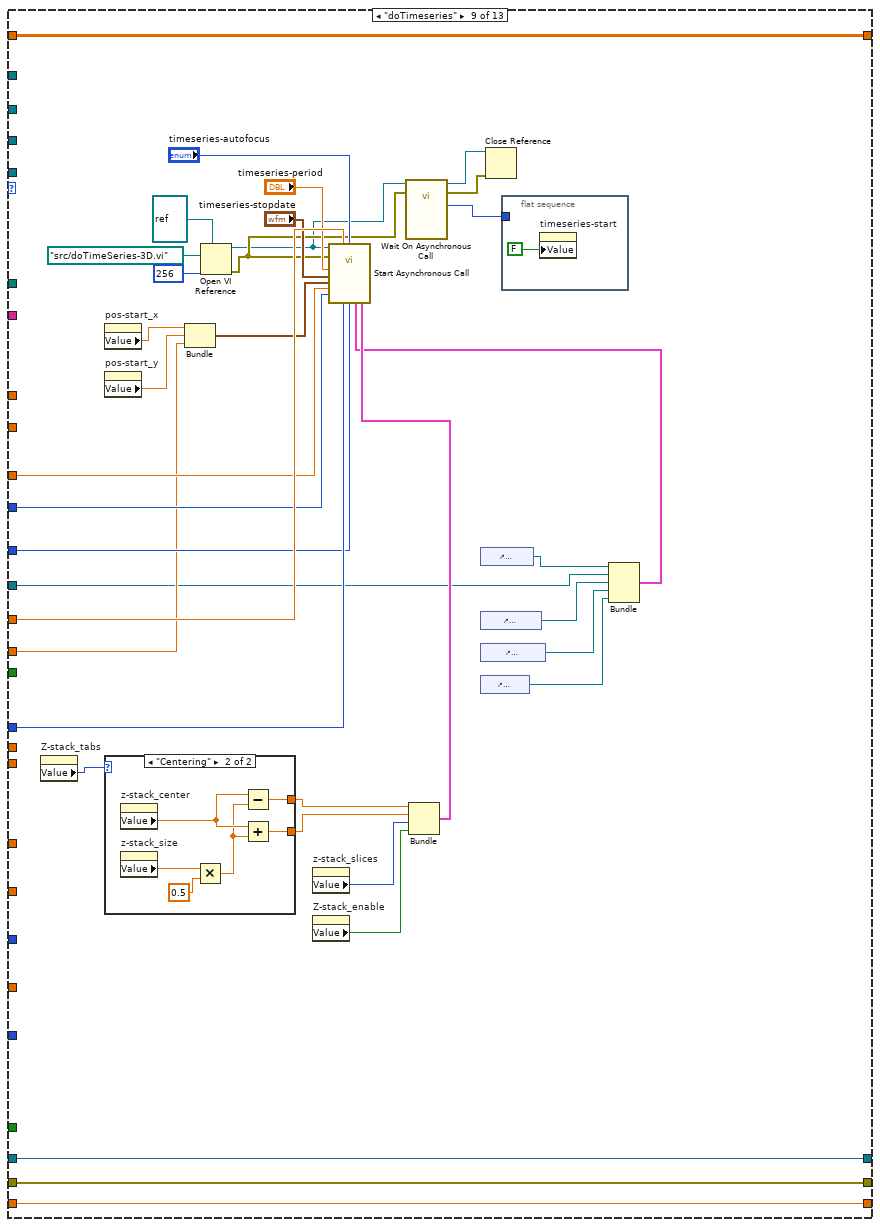
[diagram p18: hidden frame]
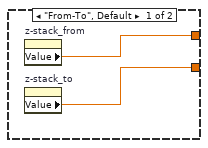
[diagram p19: hidden frame]
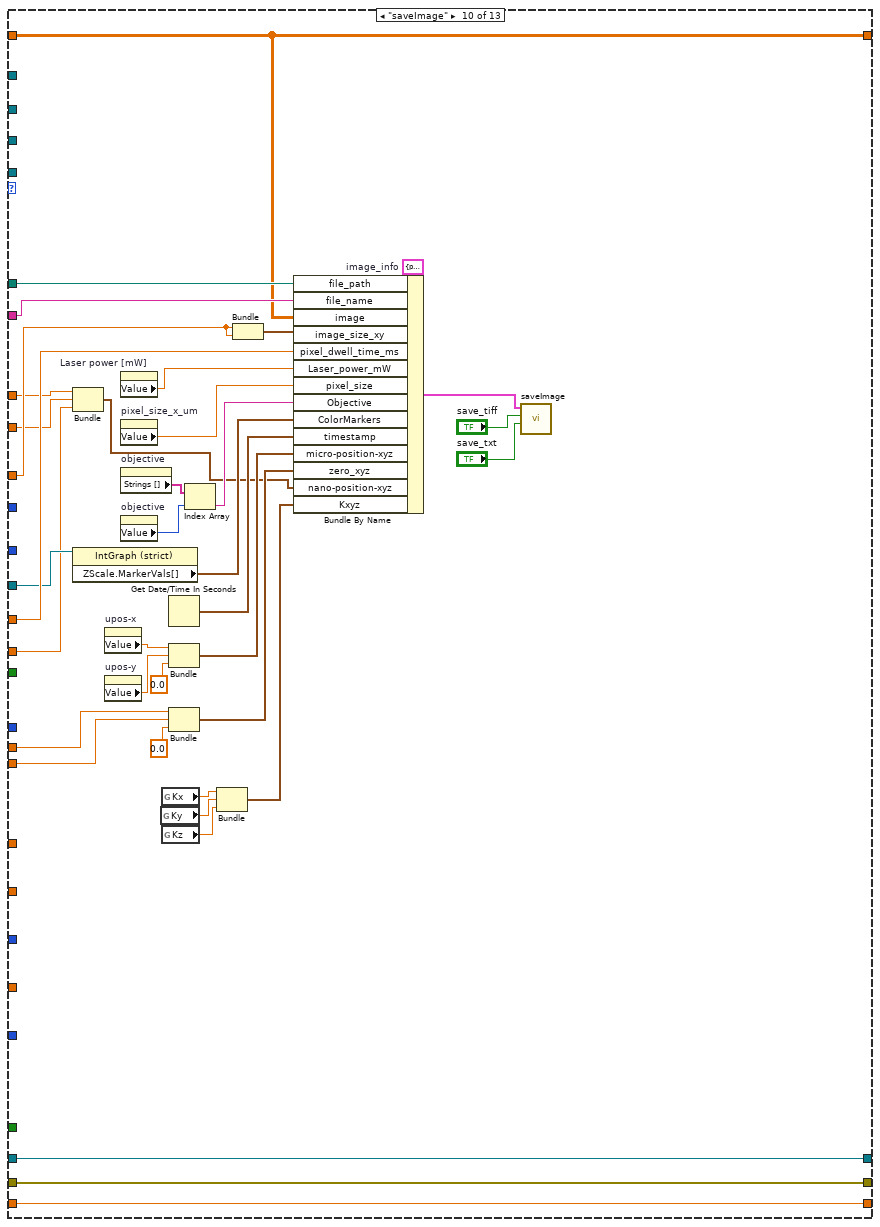
[diagram p20: hidden frame]
diagram:
  w24 = T4 {"status_x"=0.0, "status_y"=0.0, "status_z"=0.0, "pos_x"=0.0, "pos_y"=0.0, "pos_z"=0.0}  # status
  w28 = 0.0 ("upos-cpos_x")
  w29 = u32 0 ("upos-state_x")
  w30 = 0.0 ("upos-x")
  w36 = FALSE ("Cursors Scroll Graph")
  n1 = global read "GLOBAL_VAR.vi" "Motors-enable"() -> (w27:bool)
  n2 = global read "GLOBAL_VAR.vi" "Motors-enable"() -> (w17:bool)
  n3 = call <instrlib>:"PM100D Initialize.vi"("Reset Device (Reset Device)"=TRUE ("ID Query (Do Query)"), "ID Query (Do Query)"=TRUE, "resource name"=refnum<visa-resource-name> "USB0::0x1313::0x8072::P2010071::INSTR") -> ("error out"=w7:errorcluster, "instrument handle out"=w6:refnum<visa-resource-name>)  [unwired: 7 in]
  n4 = global read "GLOBAL_VAR.vi" "Motor_x_max"() -> (w35:dbl)
  n5 = global read "GLOBAL_VAR.vi" "Motor_x_min"() -> (w34:dbl)
  n6 = global read "GLOBAL_VAR.vi" "Motor_y_max"() -> (w32:dbl)
  n7 = case shown="False" w27 {
    frame False {
      n8 = property on="tile-scan_start" class="Bool (strict)"("DisabledEnum"=T7."Disabled and Grayed Out" ("Disabled")) -> ()  [unwired: 2 in, 2 out]
    }
    frame True {
      n9 = property on="tile-scan_start" class="Bool (strict)"("DisabledEnum"=T7."Enabled" ("Disabled")) -> ()  [unwired: 2 in, 2 out]
    }
  }
  n10 = global read "GLOBAL_VAR.vi" "Motor_y_min"() -> (w33:dbl)
  n11 = global read "GLOBAL_VAR.vi" "Z_max_v"() -> (w43:dbl)
  n12 = global read "GLOBAL_VAR.vi" "Z_max_um"() -> (w14:dbl)
  n13 = global read "GLOBAL_VAR.vi" "Z_min_v"() -> (w40:dbl)
  n14 = Obtain Queue(name (unnamed)="commands", element data type=T5 {enum."standby", 0.0, 0.0, 0.0}) -> (queue out=w18:refnum<queue>)  [unwired: 3 in, 2 out]
  n15 = global read "GLOBAL_VAR.vi" "Kz"() -> (w42:dbl)
  n16 = global read "GLOBAL_VAR.vi" "Kz"() -> (w39:dbl)
  n17 = Create User Event(user event datatype=w24) -> (user event=w16:refnum<user-event>, error out=w23:errorcluster)  [unwired: 1 in]
  n18 = case shown="False" w17 {
    tunnel: w16 -> [w46 w47]
    tunnel: w18 -> [_ w48]
    tunnel: [w46 w47] -> w15
    frame False {
    }
    frame True {
      n19 = call "tra25cc_driver.vi"("user_event-status_in"=w47, "queue-commands"=w48) -> ()  [unwired: 9 in, 1 out]
    }
  }
  n20 = property on="upos-x" class="DigNum (strict)"("Value"=w30) -> ()  [unwired: 2 in, 2 out]
  n21 = property on="upos-state_x" class="DigNum (strict)"("Value"=w29) -> ()  [unwired: 2 in, 2 out]
  n22 = property on="upos-cpos_x" class="DigNum (strict)"("Value"=w28) -> ()  [unwired: 2 in, 2 out]
  n23 = call <instrlib>:"PM100D Set Wavelength.vi"("error in (no error)"=w7, "Wavelength (0.0)"=561.0, "instrument handle"=w6) -> ("error out"=w12:errorcluster, "instrument handle out"=w13:refnum<visa-resource-name>)  [unwired: 7 in]
  n24 = global read "GLOBAL_VAR.vi" "Ky_oil"() -> (w1:dbl)
  n25 = global read "GLOBAL_VAR.vi" "Kx_oil"() -> (w2:dbl)
  n26 = Divide(x=w43, y=w42) -> (x/y=w41:dbl)
  n27 = Divide(x=w40, y=w39) -> (x/y=w38:dbl)
  n28 = register-events(error in=w23, w16) -> (reference out=w22:refnum<event-registration>)  [unwired: 1 in, 1 out]
  n29 = property on="scan_image" class="IntGraph (strict)"("CrsrsScrollGrph"=w36) -> ()  [unwired: 2 in, 2 out]
  n30 = property on="upos-xy_control" class="XYGraph (strict)"("CursorsScrollGraph"=w36) -> ()  [unwired: 2 in, 2 out]
  n31 = property on="pos_z" class="Slide (strict)"("Scale.Maximum"=w41, "Scale.Minimum"=w38) -> ()  [unwired: 2 in, 2 out]
  n32 = property on="upos-x" class="DigNum (strict)"("Maximum"=w35, "Minimum"=w34) -> ()  [unwired: 2 in, 2 out]
  n33 = property on="upos-xy_control" class="XYGraph (strict)"("XScale.Maximum"=w35, "XScale.Minimum"=w34, "Cursor.Cursor Position"=T6 {"X"=0.0, "Y"=0.0}, "YScale.Maximum"=w32, "YScale.Minimum"=w33) -> ()  [unwired: 2 in, 2 out]
  n34 = property on="upos-y" class="DigNum (strict)"("Maximum"=w32, "Minimum"=w33) -> ()  [unwired: 2 in, 2 out]
  n35 = property on="upos-y" class="DigNum (strict)"("Value"=w30) -> ()  [unwired: 2 in, 2 out]
  n36 = property on="upos-state_y" class="DigNum (strict)"("Value"=w29) -> ()  [unwired: 2 in, 2 out]
  n37 = property on="upos-cpos_y" class="DigNum (strict)"("Value"=w28) -> ()  [unwired: 2 in, 2 out]
  n38 = property on="focus_z" class="DigNum (strict)"("Maximum"=w14) -> ()  [unwired: 2 in, 2 out]
  n39 = global write "GLOBAL_VAR.vi" "Kx"(w2) -> ()
  n40 = global write "GLOBAL_VAR.vi" "Ky"(w1) -> ()
  n41 = while {
    shift-right: [w85] -> _
    shift-left: dbl[][][] [] ("image_out") -> [w84]
    tunnel: w22 -> [w74]
    tunnel: [w71] -> w21
    shift-right: [w70] -> w19
    shift-left: w18 -> [w72]
    tunnel: w12 -> [w61]
    tunnel: [w59] -> w11
    shift-right: [w52] -> _
    shift-left: 0.0 ("upper limit") -> [w51]
    shift-right: [w60] -> w10
    shift-left: w13 -> [w62]
    stop <- "stop" stop-if-true
    n42 = event shown="[31] \"T1_open\": Value Change" {
      selector: w74 -> [_ _ _ _ _ _ _ _ _ _ _ _ _ _ _ _ _ _ _ _ _ _ _ _ _ _ _ _ _ _ _ _ _ _ _]
      dyn-events: [_ _ _ _ _ _ _ _ _ _ _ _ _ _ _ _ _ _ _ _ _ _ _ _ _ _ _ _ _ _ _ _ _ _ _] -> w71
      timeout: 100 -> [_ _ _ _ _ _ _ _ _ _ _ _ _ _ _ _ _ _ _ _ _ _ _ _ _ _ _ _ _ _ _ _ _ _ _]
      tunnel: [T12."Standby" w528 w533 w534 w541 T15."Standby" T13."Standby" T15."Standby" T13."Standby" T13."Standby" T13."Standby" T16."Standby" T12."Standby" T12."Standby" T12."Standby" T12."Standby" T17."changeZslice" T17."Standby" w608 w615 w620 T16."Standby" T16."doRecenter" T16."Standby" T16."Standby" T16."Standby" _ _ _ _ _ w719 w723 w731 w733] -> w86
      tunnel: w72 -> [w522 w524 w529 w538 w539 w544 w548 w551 w565 w574 w577 w581 w584 w587 w590 w593 w598 w600 w604 w609 w616 w632 w641 w646 w660 w669 w677 w687 w692 w700 w715 w721 w722 w727 w732]
      tunnel: [w522 w524 w529 w538 w539 w544 w548 w551 w565 w574 w577 w581 w584 w587 w590 w593 w598 w600 w604 w609 w616 w628 w640 w646 w661 w668 w678 w687 w691 w700 w715 w721 w722 w727 w732] -> w70
      event Timeout {
        n43 = event-data() -> ()  [unwired: 1 in, 1 out]
      }
      event "scan_start": Value Change {
        n44 = event-data() -> ("NewVal"=w526:bool)  [unwired: 1 in]
        n45 = Select(t=T12."do3DScan", s=w526, f=enum16{"Standby", "doScan"}."Standby") -> (s? t:f=w528:T12)
      }
      event "live-scan": Value Change {
        n46 = event-data() -> ("NewVal"=w532:bool)  [unwired: 1 in]
        n47 = Select(t=T13."doLiveScan", s=w532, f=T13."Standby") -> (s? t:f=w533:T13)
      }
      event "counting_start": Value Change {
        n48 = event-data() -> ("NewVal"=w537:bool)  [unwired: 1 in]
        n49 = Select(t=T14."doCount", s=w537, f=T14."Standby") -> (s? t:f=w534:T14)
      }
      event "focus_start": Value Change {
        n50 = event-data() -> ("NewVal"=w540:bool)  [unwired: 1 in]
        n51 = Select(t=T15."doFocus", s=w540, f=T15."doFocus") -> (s? t:f=w541:T15)
      }
      event "pos-start_cursor": Value Change {
        n52 = event-data() -> ()  [unwired: 1 in, 1 out]
        n53 = property on="scan_image" class="IntGraph (strict)"() -> ("Cursor.Cursor X"=w547:dbl, "Cursor.Cursor Y"=w546:dbl)  [unwired: 2 in, 2 out]
        n54 = property on="pos-start_x" class="DigNum (strict)"("Value"=w547) -> ()  [unwired: 2 in, 2 out]
        n55 = property on="pos-start_y" class="DigNum (strict)"("Value"=w546) -> ()  [unwired: 2 in, 2 out]
      }
      event "pos-zero": Value Change {
        w550 = 0.0 ("pos-start_x")
        n56 = event-data() -> ()  [unwired: 1 in, 1 out]
        n57 = property on="pos-start_x" class="DigNum (strict)"("Value"=w550) -> ()  [unwired: 2 in, 2 out]
        n58 = property on="pos-start_y" class="DigNum (strict)"("Value"=w550) -> ()  [unwired: 2 in, 2 out]
      }
      event "cursor-reset": Value Change {
        n59 = event-data() -> ()  [unwired: 1 in, 1 out]
        n60 = property on="scan_image" class="IntGraph (strict)"() -> ("XScale.Maximum"=w563:dbl, "XScale.Minimum"=w558:dbl, "YScale.Maximum"=w554:dbl, "YScale.Minimum"=w553:dbl)  [unwired: 2 in, 2 out]
        n61 = Subtract(x=w563, y=w558) -> (x-y=w561:dbl)
        n62 = Subtract(x=w554, y=w553) -> (x-y=w557:dbl)
        n63 = Multiply(x=0.5 ("y"), y=w561) -> (x*y=w559:dbl)
        n64 = Multiply(x=0.5 ("y"), y=w557) -> (x*y=w555:dbl)
        n65 = Add(x=w559, y=w558) -> (x+y=w562:dbl)
        n66 = Add(x=w555, y=w553) -> (x+y=w552:dbl)
        n67 = property on="scan_image" class="IntGraph (strict)"("Cursor.Cursor X"=w562, "Cursor.Cursor Y"=w552) -> ()  [unwired: 2 in, 2 out]
      }
      event "objective": Value Change {
        n68 = event-data() -> ("NewVal"=w567:u16)  [unwired: 1 in]
        n69 = case shown="2" w567 {
          frame 0, Default {
            # "In this case, all distances\nare shown in volts."
            n70 = global read "GLOBAL_VAR.vi" "Kx_volt"() -> (w569:dbl)
            n71 = global read "GLOBAL_VAR.vi" "Ky_volt"() -> (w568:dbl)
            n72 = global write "GLOBAL_VAR.vi" "Kx"(w569) -> ()
            n73 = global write "GLOBAL_VAR.vi" "Ky"(w568) -> ()
          }
          frame 1 {
            # "100x"
            n74 = global read "GLOBAL_VAR.vi" "Kx_oil"() -> (w571:dbl)
            n75 = global read "GLOBAL_VAR.vi" "Ky_oil"() -> (w570:dbl)
            n76 = global write "GLOBAL_VAR.vi" "Kx"(w571) -> ()
            n77 = global write "GLOBAL_VAR.vi" "Ky"(w570) -> ()
          }
          frame 2 {
            n78 = global read "GLOBAL_VAR.vi" "Kx_air"() -> (w573:dbl)
            n79 = global read "GLOBAL_VAR.vi" "Ky_air"() -> (w572:dbl)
            n80 = global write "GLOBAL_VAR.vi" "Kx"(w573) -> ()
            n81 = global write "GLOBAL_VAR.vi" "Ky"(w572) -> ()
          }
        }
      }
      event "pos_z": Value Change {
        n82 = event-data() -> ("NewVal"=w575:dbl)  [unwired: 1 in]
        n83 = call "set_z.vi"("z_value_um"=w575) -> ()  [unwired: 10 in, 1 out]
        n84 = property on="focus_z" class="DigNum (strict)"("Value"=w575) -> ()  [unwired: 2 in, 2 out]
        n85 = property on="current_z" class="DigNum (strict)"("Value"=w575) -> ()  [unwired: 2 in, 2 out]
      }
      event "focus_z": Value Change {
        n86 = event-data() -> ("NewVal"=w578:dbl)  [unwired: 1 in]
        n87 = call "set_z.vi"("z_value_um"=w578) -> ()  [unwired: 10 in, 1 out]
        n88 = property on="pos_z" class="Slide (strict)"("Value"=w578) -> ()  [unwired: 2 in, 2 out]
        n89 = property on="current_z" class="DigNum (strict)"("Value"=w578) -> ()  [unwired: 2 in, 2 out]
      }
      event "focus_z_start", "focus_z_end": Value Change {
        n90 = event-data() -> ()  [unwired: 1 in, 1 out]
        n91 = property on="focus_z_end" class="DigNum (strict)"() -> ("Value"=w583:dbl)  [unwired: 2 in, 2 out]
        n92 = property on="focus_z_start" class="DigNum (strict)"() -> ("Value"=w582:dbl)  [unwired: 2 in, 2 out]
        n93 = property on="pos_z" class="Slide (strict)"("Scale.Maximum"=w583, "Scale.Minimum"=w582) -> ()  [unwired: 2 in, 2 out]
      }
      event "z-stack-set_from": Value Change {
        n94 = event-data() -> ()  [unwired: 1 in, 1 out]
        n95 = property on="current_z" class="DigNum (strict)"() -> ("Value"=w586:dbl)  [unwired: 2 in, 2 out]
        n96 = property on="z-stack_from" class="DigNum (strict)"("Value"=w586) -> ()  [unwired: 2 in, 2 out]
      }
      event "z-stack-set_to": Value Change {
        n97 = event-data() -> ()  [unwired: 1 in, 1 out]
        n98 = property on="current_z" class="DigNum (strict)"() -> ("Value"=w589:dbl)  [unwired: 2 in, 2 out]
        n99 = property on="z-stack_to" class="DigNum (strict)"("Value"=w589) -> ()  [unwired: 2 in, 2 out]
      }
      event "z-stack-set_center": Value Change {
        n100 = event-data() -> ()  [unwired: 1 in, 1 out]
        n101 = property on="current_z" class="DigNum (strict)"() -> ("Value"=w592:dbl)  [unwired: 2 in, 2 out]
        n102 = property on="z-stack_center" class="DigNum (strict)"("Value"=w592) -> ()  [unwired: 2 in, 2 out]
      }
      event "current_x", "current_y", "current_z": Value Change {
        n103 = event-data() -> ()  [unwired: 1 in, 1 out]
        n104 = call "set_xy.vi"("y_value_um"="current_y", "x_value_um"="current_x") -> ()  [unwired: 9 in, 1 out]
        n105 = call "set_z.vi"("z_value_um"="current_z") -> ()  [unwired: 10 in, 1 out]
      }
      event "z-stack_pos": Value Change {
        n106 = event-data() -> ()  [unwired: 1 in, 1 out]
      }
      event "z-stack_slices": Value Change {
        n107 = event-data() -> ("NewVal"=w603:i32)  [unwired: 1 in]
        n108 = property on="z-stack_pos" class="Slide (strict)"("Scale.Maximum"=w603, "Scale.Minimum"=1.0 ("Scale.Range:Minimum")) -> ()  [unwired: 2 in, 2 out]
      }
      event "esr_start": Value Change {
        n109 = event-data() -> ("NewVal"=w606:bool)  [unwired: 1 in]
        n110 = Select(t=T18."doESR", s=w606, f=T18."Standby") -> (s? t:f=w608:T18)
      }
      event "tile-scan_start": Value Change {
        n111 = event-data() -> ("NewVal"=w612:bool)  [unwired: 1 in]
        n112 = global read "GLOBAL_VAR.vi" "Motors-enable"() -> (w610:bool)
        n113 = And(x=w612, y=w610) -> (x .and. y?=w611:bool)
        n114 = Select(t=T19."doTileScan", s=w611, f=T19."Standby") -> (s? t:f=w615:T19)
      }
      event "timeseries-start": Value Change {
        n115 = event-data() -> ("NewVal"=w619:bool)  [unwired: 1 in]
        n116 = Select(t=T14."doTimeseries", s=w619, f=T14."Standby") -> (s? t:f=w620:T14)
      }
      event "upos-x", "upos-y": Value Change {
        n117 = event-data() -> ()  [unwired: 1 in, 1 out]
        n118 = property on="upos-x" class="DigNum (strict)"() -> ("Value"=w625:dbl)  [unwired: 2 in, 2 out]
        n119 = property on="upos-y" class="DigNum (strict)"() -> ("Value"=w624:dbl)  [unwired: 2 in, 2 out]
        n120 = property on="X Zero" class="DigNum (strict)"() -> ("Value"=w623:dbl)  [unwired: 2 in, 2 out]
        n121 = property on="Y Zero" class="DigNum (strict)"() -> ("Value"=w622:dbl)  [unwired: 2 in, 2 out]
        n122 = Subtract(x=w624, y=w622) -> (x-y=w627:dbl)
        n123 = Bundle(T20."domove", "Value"=w625, "Value"=w624, "Value"=0.0) -> (w630:T24)  [unwired: 1 in]
        n124 = Subtract(x=w625, y=w623) -> (x-y=w626:dbl)
        n125 = Enqueue Element(queue=w632, element=w630) -> (queue out=w628:refnum<queue>)  [unwired: 2 in, 2 out]
        n126 = property on="upos-xy_control" class="XYGraph (strict)"("Cursor.Cursor X"=w625, "Cursor.Cursor Y"=w624) -> ()  [unwired: 2 in, 2 out]
        n127 = property on="X Rel" class="DigNum (strict)"("Value"=w626) -> ()  [unwired: 2 in, 2 out]
        n128 = property on="Y Rel" class="DigNum (strict)"("Value"=w627) -> ()  [unwired: 2 in, 2 out]
      }
      event "X Rel", "Y Rel": Value Change {
        n129 = event-data() -> ()  [unwired: 1 in, 1 out]
        n130 = property on="X Rel" class="DigNum (strict)"() -> ("Value"=w639:dbl)  [unwired: 2 in, 2 out]
        n131 = property on="X Zero" class="DigNum (strict)"() -> ("Value"=w637:dbl)  [unwired: 2 in, 2 out]
        n132 = property on="Y Rel" class="DigNum (strict)"() -> ("Value"=w638:dbl)  [unwired: 2 in, 2 out]
        n133 = property on="Y Zero" class="DigNum (strict)"() -> ("Value"=w636:dbl)  [unwired: 2 in, 2 out]
        n134 = Add(x=w639, y=w637) -> (x+y=w635:dbl)
        n135 = Add(x=w638, y=w636) -> (x+y=w634:dbl)
        n136 = Bundle(T20."domove", w635, w634, "Value"=0.0) -> (w644:T25)  [unwired: 1 in]
        n137 = property on="upos-x" class="DigNum (strict)"("Value"=w635) -> ()  [unwired: 2 in, 2 out]
        n138 = property on="upos-y" class="DigNum (strict)"("Value"=w634) -> ()  [unwired: 2 in, 2 out]
        n139 = Enqueue Element(queue=w641, element=w644) -> (queue out=w640:refnum<queue>)  [unwired: 2 in, 2 out]
        n140 = property on="upos-xy_control" class="XYGraph (strict)"("Cursor.Cursor X"=w635, "Cursor.Cursor Y"=w634) -> ()  [unwired: 2 in, 2 out]
      }
      event "X Zero", "Y Zero": Value Change {
        n141 = event-data() -> ()  [unwired: 1 in, 1 out]
        n142 = property on="upos-x" class="DigNum (strict)"() -> ("Value"=w652:dbl)  [unwired: 2 in, 2 out]
        n143 = property on="X Zero" class="DigNum (strict)"() -> ("Value"=w648:dbl)  [unwired: 2 in, 2 out]
        n144 = property on="upos-y" class="DigNum (strict)"() -> ("Value"=w651:dbl)  [unwired: 2 in, 2 out]
        n145 = property on="Y Zero" class="DigNum (strict)"() -> ("Value"=w647:dbl)  [unwired: 2 in, 2 out]
        n146 = Subtract(x=w652, y=w648) -> (x-y=w650:dbl)
        n147 = Subtract(x=w651, y=w647) -> (x-y=w649:dbl)
        n148 = property on="X Rel" class="DigNum (strict)"("Value"=w650) -> ()  [unwired: 2 in, 2 out]
        n149 = property on="Y Rel" class="DigNum (strict)"("Value"=w649) -> ()  [unwired: 2 in, 2 out]
      }
      event "upos-xy_control": Cursor Move {
        n150 = event-data() -> ("CursLoc.X"=w659:dbl, "CursLoc.Y"=w658:dbl)  [unwired: 1 in]
        n151 = property on="X Zero" class="DigNum (strict)"() -> ("Value"=w655:dbl)  [unwired: 2 in, 2 out]
        n152 = property on="Y Zero" class="DigNum (strict)"() -> ("Value"=w654:dbl)  [unwired: 2 in, 2 out]
        n153 = property on="upos-x" class="DigNum (strict)"("Value"=w659) -> ()  [unwired: 2 in, 2 out]
        n154 = property on="upos-y" class="DigNum (strict)"("Value"=w658) -> ()  [unwired: 2 in, 2 out]
        n155 = Subtract(x=w659, y=w655) -> (x-y=w657:dbl)
        n156 = Subtract(x=w658, y=w654) -> (x-y=w656:dbl)
        n157 = Bundle(enum16{"standby", "domove", "dostop"}."standby", "X"=w659, "Y"=w658, 0.0) -> (w662:T26)  [unwired: 1 in]
        n158 = Enqueue Element(queue=w660, element=w662) -> (queue out=w661:refnum<queue>)  [unwired: 2 in, 2 out]
        n159 = property on="X Rel" class="DigNum (strict)"("Value"=w657) -> ()  [unwired: 2 in, 2 out]
        n160 = property on="Y Rel" class="DigNum (strict)"("Value"=w656) -> ()  [unwired: 2 in, 2 out]
      }
      event "upos-xy_control": Cursor Release {
        n161 = event-data() -> ()  [unwired: 1 in, 1 out]
        n162 = Bundle(enum16{"standby", "domove", "dostop", "exit"}."domove", "upos-x"="upos-x", "upos-y"="upos-y", 0.0) -> (w670:T27)  [unwired: 1 in]
        n163 = Enqueue Element(queue=w669, element=w670) -> (queue out=w668:refnum<queue>)  [unwired: 2 in, 2 out]
      }
      event "upos-stop": Value Change {
        n164 = event-data() -> ("NewVal"=w682:bool)  [unwired: 1 in]
        n165 = Select(t=enum16{"standby", "domove", "dostop", "exit"}."dostop", s=w682, f=enum16{"standby", "domove", "dostop", "exit"}."standby") -> (s? t:f=w676:enum16{"standby", "domove", "dostop", "exit"})
        n166 = Bundle(w676, 0.0, 0.0, 0.0) -> (w675:T28)  [unwired: 1 in]
        n167 = Enqueue Element(queue=w677, element=w675) -> (queue out=w678:refnum<queue>)  [unwired: 2 in, 2 out]
      }
      event User Event {
        n168 = event-data() -> ("status_x"=→"upos-state_x":dbl, "status_y"=→"upos-state_y":dbl, "pos_x"=w685:dbl, "pos_y"=w684:dbl)  [unwired: 1 in, 2 out]
        "upos-cpos_y" <- w684
        "upos-cpos_x" <- w685
        n169 = Bundle("pos_x"=w685, "pos_y"=w684) -> (w683:cluster{"pos_x":dbl, "pos_y":dbl})  [unwired: 1 in]
        n170 = Build Array(w683) -> (w686:cluster{"pos_x":dbl, "pos_y":dbl}[])
        n171 = property on="upos-xy_control" class="XYGraph (strict)"("Value"=w686) -> ()  [unwired: 2 in, 2 out]
      }
      event "stop": Value Change {
        n172 = event-data() -> ("NewVal"=w690:bool)  [unwired: 1 in]
        n173 = Select(t=enum16{"standby", "domove", "dostop", "exit"}."exit", s=w690, f=enum16{"standby", "domove", "dostop", "exit"}."standby") -> (s? t:f=w696:enum16{"standby", "domove", "dostop", "exit"})
        n174 = Bundle(w696, 0.0, 0.0, 0.0) -> (w695:T28)  [unwired: 1 in]
        n175 = Enqueue Element(queue=w692, element=w695) -> (queue out=w691:refnum<queue>)  [unwired: 2 in, 2 out]
      }
      event "timeseries-stopdate", "timeseries-period": Value Change {
        n176 = event-data() -> ()  [unwired: 1 in, 1 out]
        n177 = property on="timeseries-stopdate" class="AbsTime (strict)"() -> ("Value"=w707:timestamp)  [unwired: 2 in, 2 out]
        n178 = Get Date/Time In Seconds() -> (seconds since 1Jan1904=w706:timestamp)
        n179 = Subtract(x=w707, y=w706) -> (x-y=w705:dbl)
        n180 = Greater Than 0?(x=w705) -> (x > 0?=w704:bool)
        n181 = case shown="True" w704 {
          tunnel: w705 -> [_ w713]
          tunnel: [0.0 w711] -> w703
          tunnel: ["00:00:00" ("HH:MM:SS") w710] -> w702
          frame False {
          }
          frame True {
            n182 = property on="timeseries-period" class="DigNum (strict)"() -> ("Value"=w714:dbl)  [unwired: 2 in, 2 out]
            n183 = Divide(x=w713, y=w714) -> (x/y=w712:dbl)
            n184 = call "seconds2time.vi"("seconds"=w713) -> ("HH:MM:SS"=w710:string)  [unwired: 10 in]
            n185 = Round To Nearest(number=w712) -> (nearest integer value=w711:dbl)
          }
        }
        "timeseries-total_images" <- w703
        "timeseries-rem_time" <- w702
        "timeseries-current_image" <- 0.0 ("timeseries-current_image")
      }
      event "laser_on-off": Value Change {
        n186 = event-data() -> ("NewVal"=w716:bool)  [unwired: 1 in]
        n187 = call "laserON-OFF.vi"("ON-OFF"=w716) -> ()  [unwired: 11 in]
      }
      event "T1_open": Value Change {
        n188 = event-data() -> ("NewVal"=w720:bool)  [unwired: 1 in]
        n189 = Select(t=T21."doT1", s=w720, f=T21."Standby") -> (s? t:f=w719:T21)
      }
      event "T2_open": Value Change {
        n190 = event-data() -> ("NewVal"=w724:bool)  [unwired: 1 in]
        n191 = Select(t=T22."doT2", s=w724, f=T22."Standby") -> (s? t:f=w723:T22)
      }
      event "file_save": Value Change {
        n192 = event-data() -> ("NewVal"=w728:bool)  [unwired: 1 in]
        n193 = Select(t=T23."saveImage", s=w728, f=T23."Standby") -> (s? t:f=w731:T23)
      }
      event "recenter": Value Change {
        n194 = event-data() -> ("NewVal"=w736:bool)  [unwired: 1 in]
        n195 = Select(t=T16."doRecenter", s=w736, f=T16."Standby") -> (s? t:f=w733:T16)
      }
    }
    n196 = control-ref of="scan_image"() -> (w79:refnum<vi>)
    n197 = control-ref of="scan_start"() -> (w78:refnum<vi>)
    n198 = control-ref of="pos-start_y"() -> (w77:refnum<vi>)
    n199 = control-ref of="pos-start_x"() -> (w76:refnum<vi>)
    n200 = case shown="\"doT2\"" w86 {
      tunnel: w78 -> [_ _ _ _ w264 _ _ _ _ _ _ _ _]
      tunnel: w77 -> [_ _ _ _ _ _ _ _ _ _ _ _ _]
      tunnel: w76 -> [_ _ _ _ _ _ _ _ _ _ _ _ _]
      tunnel: [w131 w174 w195 w216 w237 w303 w334 w379 w424 w464 w476 w489 w510] -> w85
      tunnel: w84 -> [w131 w174 w195 w216 _ w303 w334 w379 w424 w464 w476 w489 w510]
      tunnel: "pixel_dwell_ms" -> [w130 _ _ _ w232 _ _ w361 w418 w461 _ _ _]
      tunnel: "scan_direction" -> [_ _ _ _ w249 _ _ w360 w411 _ _ _ _]
      tunnel: "frame_size_x_px" -> [w129 _ _ _ w233 _ _ w359 w413 _ _ _ _]
      tunnel: "pos_start" -> [_ _ _ w213 w248 _ _ w358 w412 _ _ _ _]
      tunnel: w79 -> [_ _ _ w215 w235 _ _ w357 w400 w455 _ _ _]
      tunnel: "image_size_x_um" -> [w128 _ _ w214 w234 _ _ w343 w414 w462 _ _ _]
      tunnel: w71 -> [_ _ _ _ _ _ _ w355 _ _ _ _ _]
      tunnel: w70 -> [_ _ _ _ _ _ _ w354 _ _ _ _ _]
      tunnel: "focus_z_start" -> [_ _ w194 _ _ _ _ w352 _ _ _ _ _]
      tunnel: "focus_z_end" -> [_ _ w193 _ _ _ _ w351 _ _ _ _ _]
      tunnel: "focus_q_steps" -> [_ _ w192 _ _ _ _ w350 _ _ _ _ _]
      tunnel: "focus_dwell_ms" -> [_ _ w191 _ _ _ _ w349 _ _ _ _ _]
      tunnel: "XY Max focus?" -> [_ _ _ _ _ _ _ w347 _ _ _ _ _]
      tunnel: "focus_z" -> [_ _ _ _ w240 _ w324 _ w404 w434 w471 w493 _]
      tunnel: w62 -> [w96 w168 w190 w212 w245 w299 w306 w340 w391 w470 w478 w492 w509]
      tunnel: w61 -> [w95 w167 w189 w211 w244 w298 w305 w339 w390 w469 w477 w491 w508]
      tunnel: [w94 w168 w190 w212 w245 w299 w306 w340 w391 w470 w478 w492 w509] -> w60
      tunnel: [w93 w167 w189 w211 w244 w298 w305 w339 w390 w469 w477 w491 w508] -> w59
      tunnel: "file_path" -> [_ _ _ _ w243 _ _ _ _ w466 _ _ _]
      tunnel: "file_name" -> [_ _ _ _ w242 _ _ _ _ w465 _ _ _]
      tunnel: "X Zero" -> [_ _ _ _ _ _ _ _ _ w447 _ _ _]
      tunnel: "Y Zero" -> [_ _ _ _ _ _ _ _ _ w446 _ _ _]
      tunnel: "pos-start_x" -> [_ _ _ _ w231 _ _ w337 _ w444 _ _ _]
      tunnel: "pos-start_y" -> [_ _ _ _ w230 _ _ w336 _ w443 _ _ _]
      tunnel: [w87 w166 w188 w210 w238 w297 w304 w335 w389 w435 w479 w490 w507] -> w52
      tunnel: w51 -> [_ w166 w188 w210 w238 w297 w304 w335 w389 w435 w479 w490 w507]
      tunnel: "objective" -> [_ _ _ _ w241 _ _ _ _ _ _ _ _]
      tunnel: "file_autosave" -> [_ _ _ _ w236 _ _ _ _ _ _ _ _]
      frame "Standby", Default {
        w108 = 1000.0 ("y")
        # "Power in the sample"
        # "Updates the remaining time when time series are running"
        # "Calculation of the distance between slices in a z-stack"
        # "This section shows the x-section and y-section views of the image in the the graphs"
        # "This section calculates the pixel size and the total time per image."
        n201 = property on="scan_image" class="IntGraph (strict)"() -> ("Value"=w145:dbl[][], "Cursor.Cursor X"=w138:dbl, "XScale.Offset"=w107:dbl, "XScale.Multiplier"=w127:dbl, "Cursor.Cursor Y"=w137:dbl, "YScale.Offset"=w106:dbl, "YScale.Multiplier"=w119:dbl, "Cursor.Cursor X"=w102:dbl, "Cursor.Cursor Y"=w103:dbl)  [unwired: 2 in, 2 out]
        n202 = property on="X Rel" class="DigNum (strict)"() -> ("Value"=w109:dbl)  [unwired: 2 in, 2 out]
        n203 = property on="Y Rel" class="DigNum (strict)"() -> ("Value"=w110:dbl)  [unwired: 2 in, 2 out]
        n204 = Multiply(x=w109, y=w108) -> (x*y=w100:dbl)
        n205 = Multiply(x=w110, y=w108) -> (x*y=w98:dbl)
        n206 = Square(x=w129) -> (x^2=w153:i32)
        n207 = Divide(x=w128, y=w129) -> (x/y=→"pixel_size_x_um":dbl)
        n208 = Divide(x=w128, y=w129) -> (x/y=→"pixel_size_y_um":dbl)
        n209 = Multiply(x=w153, y=w130) -> (x*y=w148:dbl)
        n210 = Add(x=w107, y=w98) -> (x+y=w105:dbl)
        n211 = Subtract(x=w138, y=w107) -> (x-y=w147:dbl)
        n212 = Subtract(x=w137, y=w106) -> (x-y=w144:dbl)
        n213 = Add(x=w106, y=w100) -> (x+y=w104:dbl)
        n214 = Add(x=w102, y=w100) -> (x+y=→"X":dbl)
        n215 = Add(x=w103, y=w98) -> (x+y=→"Y":dbl)
        n216 = Divide(x=w148, y=1000.0) -> (x/y=→"time_frame_s":dbl)
        n217 = Divide(x=w147, y=w127) -> (x/y=w146:dbl)
        n218 = Divide(x=w144, y=w119) -> (x/y=w143:dbl)
        n219 = Round To Nearest(number=w146) -> (nearest integer value=w124:dbl)
        n220 = Round To Nearest(number=w143) -> (nearest integer value=w142:dbl)
        n221 = property on="timeseries-start" class="Bool (strict)"() -> ("Value"=w97:bool)  [unwired: 2 in, 2 out]
        n222 = Index Array(array=w145, index (row)=w124) -> (element=w117:dbl[])  [unwired: 1 in]
        n223 = Index Array(array=w145, index (col)=w142) -> (element=w120:dbl[])  [unwired: 1 in]
        n224 = global read "GLOBAL_VAR.vi" "power_factor"() -> (w88:dbl)
        n225 = case shown="False" w97 {
          frame False {
          }
          frame True {
            n226 = property on="timeseries-stopdate" class="AbsTime (strict)"() -> ("Value"=w158:timestamp)  [unwired: 2 in, 2 out]
            n227 = Get Date/Time In Seconds() -> (seconds since 1Jan1904=w157:timestamp)
            n228 = Subtract(x=w158, y=w157) -> (x-y=w155:dbl)
            n229 = Greater Than 0?(x=w155) -> (x > 0?=w156:bool)
            n230 = case shown="True" w156 {
              tunnel: w155 -> [_ w161]
              tunnel: ["00:00:00" ("HH:MM:SS") w160] -> w154
              frame False {
              }
              frame True {
                n231 = call "seconds2time.vi"("seconds"=w161) -> ("HH:MM:SS"=w160:string)  [unwired: 10 in]
              }
            }
            n232 = property on="timeseries-rem_time" class="Str"("Value"=w154) -> ()  [unwired: 2 in, 2 out]
          }
        }
        n233 = property on="Z-stack_tabs" class="TabCtl (strict)"() -> ("Value"=w139:enum32{"From-To", "Centering"})  [unwired: 2 in, 2 out]
        n234 = Array Size(array=w117) -> (size(s)=w125:i32)
        n235 = Array Size(array=w120) -> (size(s)=w122:i32)
        n236 = call <instrlib>:"PM100D Measure Power.vi"("error in (no error)"=w95, "instrument handle"=w96) -> ("error out"=w93:errorcluster, "Power"=w92:dbl, "instrument handle out"=w94:refnum<visa-resource-name>)  [unwired: 7 in]
        n237 = Decrement(x=w125) -> (x-1=w112:i32)
        n238 = Decrement(x=w122) -> (x-1=w111:i32)
        n239 = case shown="\"From-To\", Default" w139 {
          tunnel: [w162 w165] -> w140
          frame "From-To", Default {
            n240 = property on="z-stack_to" class="DigNum (strict)"() -> ("Value"=w164:dbl)  [unwired: 2 in, 2 out]
            n241 = property on="z-stack_from" class="DigNum (strict)"() -> ("Value"=w163:dbl)  [unwired: 2 in, 2 out]
            n242 = Subtract(x=w164, y=w163) -> (x-y=w162:dbl)
          }
          frame "Centering" {
            n243 = property on="z-stack_size" class="DigNum (strict)"() -> ("Value"=w165:dbl)  [unwired: 2 in, 2 out]
          }
        }
        n244 = Multiply(x=w112, y=w127) -> (x*y=w126:dbl)
        n245 = Multiply(x=w111, y=w119) -> (x*y=w123:dbl)
        n246 = Multiply(x=w92, y=w88) -> (x*y=w91:dbl)
        n247 = Add(x=w126, y=w105) -> (x+y=w114:dbl)
        n248 = Add(x=w123, y=w104) -> (x+y=w113:dbl)
        n249 = property on="z-stack_slices" class="DigNum (strict)"() -> ("Value"=w141:i32)  [unwired: 2 in, 2 out]
        n250 = In Range and Coerce(upper limit=inf, x=w91, lower limit=0.0) -> (coerced(x)=w87:dbl)  [unwired: 1 out]
        "Laser power [mW]" <- w87
        n251 = call-poly <vilib>:"Ramp Pattern.vi"("start"=w105, "end"=w114, "samples"=w125) -> ("Ramp Pattern"=w118:dbl[])  [unwired: 7 in, 1 out]
        n252 = call-poly <vilib>:"Ramp Pattern.vi"("start"=w104, "end"=w113, "samples"=w122) -> ("Ramp Pattern"=w121:dbl[])  [unwired: 7 in, 1 out]
        n253 = Decrement(x=w141) -> (x-1=w132:i32)
        n254 = Bundle("Value"=w117, "Ramp Pattern"=w118) -> (→"XY Graph":cluster{"Value":dbl[], "Ramp Pattern":dbl[]})  [unwired: 1 in]
        n255 = Bundle("Ramp Pattern"=w121, "Value"=w120) -> (→"XY Graph 2":cluster{"Ramp Pattern":dbl[], "Value":dbl[]})  [unwired: 1 in]
        n256 = Divide(x=w140, y=w132) -> (x/y=w136:dbl)
        n257 = Greater Than 0?(x=w132) -> (x > 0?=w133:bool)
        n258 = property on="XY Graph" class="XYGraph (strict)"("YScale.Maximum"=w114, "YScale.Minimum"=w105) -> ()  [unwired: 2 in, 2 out]
        n259 = property on="XY Graph 2" class="XYGraph (strict)"("XScale.Maximum"=w113, "XScale.Minimum"=w104) -> ()  [unwired: 2 in, 2 out]
        n260 = Select(t=w136, s=w133, f=0.0) -> (s? t:f=→"z-stack_step_size":dbl)
        "frame_size_y_px" <- w129
        "image_size_y_um" <- w128
      }
      frame "doCount" {
        n261 = control-ref of="wavechart_01"() -> (w175:refnum<vi>)
        n262 = control-ref of="counts"() -> (w176:refnum<vi>)
        n263 = control-ref of="scan_image"() -> (w177:refnum<vi>)
        n264 = Open VI Reference(type specifier VI Refnum (for type only)=refnum<vi> refnum, vi path=path "src/doCount.vi", options=128) -> (vi reference=w182:refnum<vi>, error out=w183:errorcluster)  [unwired: 3 in]
        n265 = control-ref of="counting_start"() -> (w178:refnum<vi>)
        n266 = Multiply(x="counts_dwell_time", y=0.001) -> (x*y=w173:dbl)
        n267 = call-by-ref "Start Asynchronous Call"(reference=w182, error in=w183, "counts_out_ref_chart"=w175, "counts_out_ref"=w176, "enable"=w178, "Acquisition time [s]"=w173, "cursors_ref"=w177) -> (reference out=w184:refnum<vi>, error out=w185:errorcluster)  [unwired: 7 in]
        n268 = property on="wavechart_01" class="WFChart (strict)"("XScale.Multiplier"=1.0 ("X Scale.Offset and Multiplier:Multiplier"), "XScale.Offset"=0.0 ("X Scale.Offset and Multiplier:Offset"), "History Data"=dbl[] []) -> ()  [unwired: 2 in, 2 out]
        n269 = Close Reference(reference=w184, error in (no error)=w185) -> ()  [unwired: 1 out]
      }
      frame "doFocus" {
        n270 = property on="scan_image" class="IntGraph (strict)"() -> ("Cursor.Cursor X"=w198:dbl, "Cursor.Cursor Y"=w197:dbl)  [unwired: 2 in, 2 out]
        n271 = Decrement(x=w192) -> (x-1=w200:i32)
        n272 = Subtract(x=w193, y=w194) -> (x-y=w201:dbl)
        n273 = call "set_xy.vi"("y_value_um"=w197, "x_value_um"=w198) -> ("error out"=w187:errorcluster)  [unwired: 9 in]
        n274 = control-ref of="wavechart_01"() -> (w203:refnum<vi>)
        n275 = Divide(x=w201, y=w200) -> (x/y=w199:dbl)
        n276 = flat-sequence {
          tunnel: w203 -> [w209]
          tunnel: [w208] -> w196
          tunnel: w194 -> [w207]
          tunnel: w193 -> [w206]
          tunnel: w192 -> [w205]
          tunnel: w191 -> [w204]
          tunnel: w187 -> [_]
          frame #0 {
            n277 = call "auto_focus.vi"("counts"=w209, "dwell_time_ms"=w204, "q_steps"=w205, "z_end"=w206, "z_start"=w207) -> ("z_focus"=w208:dbl)  [unwired: 5 in, 1 out]
          }
        }
        n278 = property on="wavechart_01" class="WFChart (strict)"("History Data"=dbl[] [], "XScale.Offset"=w194, "XScale.Multiplier"=w199) -> ()  [unwired: 2 in, 2 out]
        n279 = property on="focus_z" class="DigNum (strict)"("Val(Sgnl)"=w196) -> ()  [unwired: 2 in, 2 out]
        n280 = property on="current_z" class="DigNum (strict)"("Value"=w196) -> ()  [unwired: 2 in, 2 out]
      }
      frame "doLiveScan" {
        n281 = Open VI Reference(type specifier VI Refnum (for type only)=refnum<vi> refnum, vi path=path "src/live_scanner.vi", options=128) -> (vi reference=w224:refnum<vi>, error out=w228:errorcluster)  [unwired: 3 in]
        n282 = control-ref of="live-scan"() -> (w221:refnum<vi>)
        n283 = control-ref of="pos-start_y"() -> (w222:refnum<vi>)
        n284 = control-ref of="pos-start_x"() -> (w223:refnum<vi>)
        n285 = call-by-ref "Start Asynchronous Call"(reference=w224, error in=w228, "live_pixel_dwell_ms"="live_pixel_dwell_ms", "pos-start_x"=w223, "pos-start_y"=w222, "enable"=w221, "live_frame_size_x_px"="live_frame_size_x_px", "image_size_x_um"=w214, "pos_start"=w213, "live_scan_direction"="live_scan_direction", "IntensityGraph in"=w215) -> (reference out=w227:refnum<vi>, error out=w226:errorcluster)  [unwired: 6 in, 1 out]
        n286 = Close Reference(reference=w227, error in (no error)=w226) -> ()  [unwired: 1 out]
      }
      frame "do3DScan" {
        n287 = Bundle("pos-start_x"=w231, "pos-start_y"=w230, "focus_z"=w240) -> (w239:T29)  [unwired: 1 in]
        n288 = case shown="\"Centering\"" "Z-stack_tabs" {
          tunnel: ["z-stack_from" w293] -> w260
          tunnel: ["z-stack_to" w294] -> w259
          frame "From-To", Default {
          }
          frame "Centering" {
            n289 = Multiply(x="z-stack_size", y=0.5) -> (x*y=w291:dbl)
            n290 = Subtract(x="z-stack_center", y=w291) -> (x-y=w293:dbl)
            n291 = Add(x="z-stack_center", y=w291) -> (x+y=w294:dbl)
          }
        }
        n292 = Open VI Reference(type specifier VI Refnum (for type only)=refnum<vi> refnum, vi path=path "src/3D_scanner.vi", options=256) -> (vi reference=w257:refnum<vi>, error out=w254:errorcluster)  [unwired: 3 in]
        n293 = call-by-ref "Start Asynchronous Call"(reference=w257, error in=w254, "pixel_dwell_ms"=w232, "pos-start_x"=w231, "pos-start_y"=w230, "enable"=w264, "frame_size_x_px"=w233, "image_size_x_um"=w234, "pos_start"=w248, "z-stack_enable"="Z-stack_enable", "scan_direction"=w249, "IntensityGraph in"=w235, "z_start"=w260, "z_end"=w259, "z_q_slices"="z-stack_slices") -> ()  [unwired: 2 in, 3 out]
        n294 = call-by-ref "Wait On Asynchronous Call"(reference=w257, error in=w254) -> (reference out=w256:refnum<vi>, error out=w255:errorcluster, "image_out"=w237:dbl[][][])  [unwired: 15 in]
        n295 = case shown="True" w236 {
          tunnel: w243 -> [_ w286]
          tunnel: w242 -> [_ w285]
          tunnel: w234 -> [_ w284]
          tunnel: w232 -> [_ w282]
          tunnel: w241 -> [_ w278]
          tunnel: w239 -> [_ w275]
          tunnel: w238 -> [_ w274]
          tunnel: w237 -> [_ w273]
          frame False {
          }
          frame True {
            w288 = T30 {"file_path"=path "", "file_name"="", "image"=[], "image_size_xy"={"image_size_x_um"=1.0, "image_size_y_um"=1.0}, "pixel_dwell_time_ms"=1.0, "Laser_power_mW"=1.0, "pixel_size"=0.0, "tile_ij"={"tile_i"=0, "tile_j"=0}, "Objective"="", "ColorMarkers"=[], "timestamp"=timestamp(0 s since 1904-01-01), "micro-position-xyz"={"micro-position_x_mm"=1.0, "micro-position_y_mm"=1.0, "micro-position_z_mm"=1.0}, "zero_xyz"={"zero_x_mm"=0.0, "zero_y_mm"=0.0, "zero_z_mm"=0.0}, "nano-position-xyz"={"nano-position_x_V"=1.0, "nano-position_y_V"=1.0, "nano-position_z_V"=1.0}, "Kxyz"={"Kx_V/um"=1.0, "Ky_V/um"=1.0, "Kz_V/um"=1.0}}  # image_info
            n296 = property on="scan_image" class="IntGraph (strict)"() -> ("ZScale.MarkerVals[]"=w277:cluster{dbl, u32}[])  [unwired: 2 in, 2 out]
            n297 = property on="objective" class="Ring (strict)"() -> ("Strings []"=w280:string[])  [unwired: 2 in, 2 out]
            n298 = global read "GLOBAL_VAR.vi" "Ky"() -> (w271:dbl)
            n299 = global read "GLOBAL_VAR.vi" "Kx"() -> (w270:dbl)
            n300 = global read "GLOBAL_VAR.vi" "Kz"() -> (w272:dbl)
            n301 = property on="pixel_size_x_um" class="DigNum (strict)"() -> ("Value"=w281:dbl)  [unwired: 2 in, 2 out]
            n302 = Bundle("image_size_x_um"=w284, "image_size_x_um"=w284) -> (w283:T31)  [unwired: 1 in]
            n303 = Index Array(array=w280, index=w278) -> (element=w279:string)
            n304 = Get Date/Time In Seconds() -> (seconds since 1Jan1904=w276:timestamp)
            n305 = Bundle("Kx"=w270, "Ky"=w271, "Kz"=w272) -> (w269:cluster{"Kx":dbl, "Ky":dbl, "Kz":dbl})  [unwired: 1 in]
            n306 = Bundle By Name(cluster=w288, "image"=w273, "nano-position-xyz"=w275, "file_path"=w286, "file_name"=w285, "image_size_xy"=w283, "pixel_dwell_time_ms"=w282, "pixel_size"=w281, "Objective"=w279, "ColorMarkers"=w277, "timestamp"=w276, "Kxyz"=w269, "Laser_power_mW"=w274) -> (w287:T30)
            n307 = call "saveImage.vi"("save_txt"=TRUE ("save_tiff"), "save_tiff"=TRUE, "image_info"=w287) -> ()  [unwired: 9 in]
          }
        }
        n308 = Array Size(array=w237) -> (size(s)=w253:i32[])
        n309 = Close Reference(reference=w256, error in (no error)=w255) -> ()  [unwired: 1 out]
        n310 = Index Array(array=w253, index=0) -> (element=w251:i32)
        n311 = property on="z-stack_pos" class="Slide (strict)"("Scale.Maximum"=w251, "Scale.Minimum"=1.0 ("Scale.Range:Minimum")) -> (error out=w247:errorcluster)  [unwired: 2 in, 1 out]
        n312 = property on="scan_start" class="Bool (strict)"(error in=w247, "Value"=FALSE ("scan_start")) -> ()  [unwired: 1 in, 2 out]
      }
      frame "changeZslice" {
        n313 = Decrement(x="z-stack_pos") -> (x-1=w301:i32)
        n314 = Index Array(array=w303, index (dim 0)=w301) -> (element=→"scan_image":dbl[][])  [unwired: 2 in]
      }
      frame "doESR" {
        n315 = property on="scan_image" class="IntGraph (strict)"() -> ("Cursor.Cursor X"=w326:dbl, "Cursor.Cursor Y"=w325:dbl)  [unwired: 2 in, 2 out]
        n316 = Open VI Reference(type specifier VI Refnum (for type only)=refnum<vi> refnum, vi path=path "src/ESR/doESR.vi", options=128) -> (vi reference=w331:refnum<vi>, error out=w330:errorcluster)  [unwired: 3 in]
        n317 = Bundle("esr_repetitions"="esr_repetitions", "esr_power"="esr_power", "esr_freq_start"="esr_freq_start", "esr_freq_stop"="esr_freq_stop", "esr_step_size"="esr_step_size", "esr_dwell_time"="esr_dwell_time") -> (w308:T32)  [unwired: 1 in]
        n318 = Bundle("Cursor.Cursor X"=w326, "Cursor.Cursor Y"=w325, "focus_z"=w324) -> (w323:T33)  [unwired: 1 in]
        n319 = Subtract(x="esr_freq_stop", y="esr_freq_start") -> (x-y=w317:ext)
        n320 = Divide(x=w317, y="esr_step_size") -> (x/y=w316:ext)
        n321 = Compound Arithmetic op=MULTIPLY("esr_repetitions", w316, "esr_dwell_time") -> (→"esr_total_time":ext)
        n322 = control-ref of="esr_current_run"() -> (w322:refnum<vi>)
        n323 = control-ref of="ESR_stack"() -> (w307:refnum<vi>)
        n324 = call-by-ref "Start Asynchronous Call"(reference=w331, error in=w330, "IntGraph Refnum"=w307, "current_run_ref"=w322, "generator_enable"="esr_out_enable", "sweep_parameters"=w308, "position_xyz"=w323) -> (reference out=w327:refnum<vi>, error out=w328:errorcluster)  [unwired: 7 in]
        n325 = property on="esr_repetitions" class="DigNum (strict)"() -> ("Value"=w318:i32)  [unwired: 2 in, 2 out]
        n326 = property on="esr_current_run" class="DigNum (strict)"() -> ("Value"=w319:i32)  [unwired: 2 in, 2 out]
        n327 = Close Reference(reference=w327, error in (no error)=w328) -> ()  [unwired: 1 out]
        n328 = Subtract(x=w318, y=w319) -> (x-y=→"esr_remain":i32)
        "esr_power_led" <- "esr_out_enable"
      }
      frame "doTileScan" {
        n329 = Bundle("pos-start_x"=w337, "pos-start_y"=w336) -> (w338:cluster{"pos-start_x":dbl, "pos-start_y":dbl})  [unwired: 1 in]
        n330 = Bundle By Name(cluster=T9 {"z_start"=0.0, "z_end"=0.0, "q_steps"=0, "dwell_time_ms"=0.0} ("Focus (Piezo)"), "z_start"=w352, "z_end"=w351, "q_steps"=w350, "dwell_time_ms"=w349) -> (w348:T9)
        n331 = Bundle("tile_start_x_mm"="tile_start_x_mm", "tile_start_y_mm"="tile_start_y_mm") -> (w376:T34)  [unwired: 1 in]
        n332 = Multiply(x=w376, y=1000.0 ("tile_start_y_mm")) -> (x*y=w366:T34)
        n333 = case shown="\"tiles\", Default" "tile_tiles-size" {
          tunnel: w366 -> [w383 w388]
          tunnel: [w384 w387] -> w365
          tunnel: w343 -> [w382 _]
          frame "tiles", Default {
            n334 = Decrement(x="tile_q-tiles_x") -> (x-1=w381:dbl)
            n335 = Multiply(x=w382, y=w381) -> (x*y=w385:dbl)
            n336 = Add(x=w383, y=w385) -> (x+y=w384:T34)
            "tile_q-tiles_y" <- "tile_q-tiles_x"
          }
          frame "size" {
            n337 = Add(x=w388, y="tile_size_x_um") -> (x+y=w387:T34)
            "tile_size_y_um" <- "tile_size_x_um"
          }
        }
        n338 = Bundle By Name(cluster=T10 {"image_size"=0.0, "image_xy_start"={"image-x_start"=0.0, "image-y_start"=0.0}, "pixel_dwell_ms"=0.0, "frame_size_x_px"=0, "scan_direction"=enum."0", "pos_start"=enum."bottom-left"} ("Image (mirrors)"), "image_size"=w343, "image_xy_start"=w338, "pixel_dwell_ms"=w361, "frame_size_x_px"=w359, "scan_direction"=w360, "pos_start"=w358) -> (w362:T10)
        n339 = property on="X Zero" class="DigNum (strict)"() -> ("Value"=w345:dbl)  [unwired: 2 in, 2 out]
        n340 = property on="Y Zero" class="DigNum (strict)"() -> ("Value"=w344:dbl)  [unwired: 2 in, 2 out]
        n341 = Open VI Reference(type specifier VI Refnum (for type only)=refnum<vi> refnum, vi path=path "src/doTileScan.vi", options=128) -> (vi reference=w372:refnum<vi>, error out=w369:errorcluster)  [unwired: 3 in]
        n342 = Bundle("Value"=w345, "Value"=w344) -> (w342:cluster{"Value":dbl, "Value":dbl})  [unwired: 1 in]
        n343 = Bundle By Name(cluster=T8 {"overlap"=0.0, "pos-xy_start"={"pos-x_start"=0.0, "pos-y_start"=0.0}, "pos-xy_end"={"pos-x_end"=0.0, "pos-y_end"=0.0}, "pos-xy_ref"={"pos-x_start"=0.0, "pos-y_start"=0.0}} ("Positioners (motors)"), "overlap"="tiles-overlap", "pos-xy_start"=w366, "pos-xy_end"=w365, "pos-xy_ref"=w342) -> (w341:T8)
        n344 = control-ref of="wavechart_01"() -> (w356:refnum<vi>)
        n345 = call-by-ref "Start Asynchronous Call"(reference=w372, error in=w369, "Positioners (motors)"=w341, "IntensityGraph in"=w357, "status-event"=w355, "Image (mirrors)"=w362, "Focus (Piezo)"=w348, "XY Max?"=w347, "queue-commands"=w354, "WFChart Refnum"=w356) -> (reference out=w368:refnum<vi>, error out=w367:errorcluster)  [unwired: 8 in]
        n346 = Close Reference(reference=w368, error in (no error)=w367) -> ()  [unwired: 1 out]
      }
      frame "doTimeseries" {
        n347 = property on="Z-stack_tabs" class="TabCtl (strict)"() -> ("Value"=w410:enum32{"From-To", "Centering"})  [unwired: 2 in, 2 out]
        n348 = property on="pos-start_x" class="DigNum (strict)"() -> ("Value"=w423:dbl)  [unwired: 2 in, 2 out]
        n349 = property on="pos-start_y" class="DigNum (strict)"() -> ("Value"=w422:dbl)  [unwired: 2 in, 2 out]
        n350 = case shown="\"Centering\"" w410 {
          tunnel: [w427 w429] -> w409
          tunnel: [w426 w428] -> w408
          frame "From-To", Default {
            n351 = property on="z-stack_from" class="DigNum (strict)"() -> ("Value"=w427:dbl)  [unwired: 2 in, 2 out]
            n352 = property on="z-stack_to" class="DigNum (strict)"() -> ("Value"=w426:dbl)  [unwired: 2 in, 2 out]
          }
          frame "Centering" {
            n353 = property on="z-stack_center" class="DigNum (strict)"() -> ("Value"=w433:dbl)  [unwired: 2 in, 2 out]
            n354 = property on="z-stack_size" class="DigNum (strict)"() -> ("Value"=w432:dbl)  [unwired: 2 in, 2 out]
            n355 = Multiply(x=w432, y=0.5) -> (x*y=w431:dbl)
            n356 = Subtract(x=w433, y=w431) -> (x-y=w429:dbl)
            n357 = Add(x=w433, y=w431) -> (x+y=w428:dbl)
          }
        }
        n358 = Bundle("Value"=w423, "Value"=w422, "focus_z"=w404) -> (w415:cluster{"Value":dbl, "Value":dbl, "focus_z":dbl})  [unwired: 1 in]
        n359 = Open VI Reference(type specifier VI Refnum (for type only)=refnum<vi> refnum, vi path=path "src/doTimeSeries-3D.vi", options=256) -> (vi reference=w395:refnum<vi>, error out=w396:errorcluster)  [unwired: 3 in]
        n360 = property on="z-stack_slices" class="DigNum (strict)"() -> ("Value"=w407:i32)  [unwired: 2 in, 2 out]
        n361 = property on="Z-stack_enable" class="Bool (strict)"() -> ("Value"=w406:bool)  [unwired: 2 in, 2 out]
        n362 = call-by-ref "Wait On Asynchronous Call"(reference=w395, error in=w396) -> (reference out=w394:refnum<vi>, error out=w393:errorcluster, "return"=w392:enum16{"Error", "OK"})  [unwired: 15 in]
        n363 = Bundle("Value"=w409, "Value"=w408, "Value"=w407, "Value"=w406) -> (w405:T35)  [unwired: 1 in]
        n364 = control-ref of="timeseries-current_image"() -> (w398:refnum<vi>)
        n365 = control-ref of="timeseries-start"() -> (w401:refnum<vi>)
        n366 = control-ref of="timeseries-next_scan"() -> (w399:refnum<vi>)
        n367 = control-ref of="timeseries-rem_time"() -> (w397:refnum<vi>)
        n368 = Close Reference(reference=w394, error in (no error)=w393) -> ()  [unwired: 1 out]
        n369 = flat-sequence {
          tunnel: w392 -> [_]
          frame #0 {
            n370 = property on="timeseries-start" class="Bool (strict)"("Value"=FALSE ("timeseries-start")) -> ()  [unwired: 2 in, 2 out]
          }
        }
        n371 = Bundle("timeseries-current_image"=w398, "scan_image"=w400, "timeseries-start"=w401, "timeseries-next_scan"=w399, "timeseries-rem_time"=w397) -> (w402:T36)  [unwired: 1 in]
        n372 = call-by-ref "Start Asynchronous Call"(reference=w395, error in=w396, "period_s"="timeseries-period", "pixel_dwell_ms"=w418, "timeseries-autofocus"="timeseries-autofocus", "date_stop"="timeseries-stopdate", "pos_start_xyz"=w415, "image_size_x_um"=w414, "frame_size_x_px"=w413, "pos_start"=w412, "scan_direction"=w411, "GUI_references"=w402, "z-stack_parameters"=w405) -> ()  [unwired: 4 in, 3 out]
      }
      frame "saveImage" {
        w468 = T30 {"file_path"=path "", "file_name"="", "image"=[], "image_size_xy"={"image_size_x_um"=1.0, "image_size_y_um"=1.0}, "pixel_dwell_time_ms"=1.0, "Laser_power_mW"=1.0, "pixel_size"=0.0, "tile_ij"={"tile_i"=0, "tile_j"=0}, "Objective"="", "ColorMarkers"=[], "timestamp"=timestamp(0 s since 1904-01-01), "micro-position-xyz"={"micro-position_x_mm"=1.0, "micro-position_y_mm"=1.0, "micro-position_z_mm"=1.0}, "zero_xyz"={"zero_x_mm"=0.0, "zero_y_mm"=0.0, "zero_z_mm"=0.0}, "nano-position-xyz"={"nano-position_x_V"=1.0, "nano-position_y_V"=1.0, "nano-position_z_V"=1.0}, "Kxyz"={"Kx_V/um"=1.0, "Ky_V/um"=1.0, "Kz_V/um"=1.0}}  # image_info
        n373 = Bundle("pos-start_x"=w444, "pos-start_y"=w443, "focus_z"=w434) -> (w442:T29)  [unwired: 1 in]
        n374 = property class="IntGraph (strict)"(reference=w455) -> ("ZScale.MarkerVals[]"=w454:cluster{dbl, u32}[])  [unwired: 1 in, 2 out]
        n375 = property on="upos-x" class="DigNum (strict)"() -> ("Value"=w452:dbl)  [unwired: 2 in, 2 out]
        n376 = property on="upos-y" class="DigNum (strict)"() -> ("Value"=w451:dbl)  [unwired: 2 in, 2 out]
        n377 = property on="Laser power [mW]" class="DigNum (strict)"() -> ("Value"=w460:dbl)  [unwired: 2 in, 2 out]
        n378 = property on="pixel_size_x_um" class="DigNum (strict)"() -> ("Value"=w459:dbl)  [unwired: 2 in, 2 out]
        n379 = property on="objective" class="Ring (strict)"() -> ("Strings []"=w458:string[])  [unwired: 2 in, 2 out]
        n380 = property on="objective" class="Ring (strict)"() -> ("Value"=w457:u16)  [unwired: 2 in, 2 out]
        n381 = global read "GLOBAL_VAR.vi" "Ky"() -> (w440:dbl)
        n382 = global read "GLOBAL_VAR.vi" "Kx"() -> (w441:dbl)
        n383 = global read "GLOBAL_VAR.vi" "Kz"() -> (w439:dbl)
        n384 = Get Date/Time In Seconds() -> (seconds since 1Jan1904=w453:timestamp)
        n385 = Bundle("Value"=w452, "Value"=w451, "upos-y"=0.0) -> (w449:cluster{"Value":dbl, "Value":dbl, "upos-y":dbl})  [unwired: 1 in]
        n386 = Bundle("X Zero"=w447, "Y Zero"=w446, "upos-y"=0.0) -> (w445:T37)  [unwired: 1 in]
        n387 = Index Array(array=w458, index=w457) -> (element=w456:string)
        n388 = Bundle("Kx"=w441, "Ky"=w440, "Kz"=w439) -> (w438:cluster{"Kx":dbl, "Ky":dbl, "Kz":dbl})  [unwired: 1 in]
        n389 = Bundle("image_size_x_um"=w462, "image_size_x_um"=w462) -> (w463:T31)  [unwired: 1 in]
        n390 = Bundle By Name(cluster=w468, "file_path"=w466, "file_name"=w465, "image"=w464, "image_size_xy"=w463, "pixel_dwell_time_ms"=w461, "Laser_power_mW"=w460, "pixel_size"=w459, "Objective"=w456, "ColorMarkers"=w454, "timestamp"=w453, "micro-position-xyz"=w449, "zero_xyz"=w445, "nano-position-xyz"=w442, "Kxyz"=w438) -> (w467:T30)
        n391 = call "saveImage.vi"("save_txt"="save_txt", "save_tiff"="save_tiff", "image_info"=w467) -> ()  [unwired: 9 in]
      }
      frame "doT1" {
        n392 = property on="scan_image" class="IntGraph (strict)"() -> ("Cursor.Cursor X"=w474:dbl, "Cursor.Cursor Y"=w473:dbl)  [unwired: 2 in, 2 out]
        n393 = Bundle By Name(cluster=T11 {"nano-position_X_um"=0.0, "nano-position_Y_um"=0.0, "nano-position Z_um"=0.0} ("input_xyz"), "nano-position_X_um"=w474, "nano-position_Y_um"=w473, "nano-position Z_um"=w471) -> (w472:T11)
        n394 = flat-sequence {
          tunnel: path "C:/SpinCore/SpinAPI/lib/spinapi64.dll" ("path in") -> [w485]
          tunnel: [w484] -> w482
          tunnel: [w483] -> w481
          tunnel: w482 -> [_]
          tunnel: w481 -> [_]
          tunnel: w472 -> [w487]
          frame #0 {
            n395 = call "pb-stop.vi"("path in"=w485) -> ("error out"=w483:errorcluster, "path out"=w484:path)  [unwired: 9 in]
            n396 = Wait (ms)(milliseconds to wait=u32 100) -> ()  [unwired: 1 out]
          }
          frame #1 {
            n397 = call "gui_T1.vi"("input_xyz"=w487) -> ()  [unwired: 11 in]
            n398 = property on="laser_on-off" class="Bool (strict)"("Value"=FALSE ("laser_on-off")) -> ()  [unwired: 2 in, 2 out]
          }
        }
      }
      frame "doT2" {
        n399 = property on="scan_image" class="IntGraph (strict)"() -> ("Cursor.Cursor X"=w496:dbl, "Cursor.Cursor Y"=w495:dbl)  [unwired: 2 in, 2 out]
        n400 = Bundle By Name(cluster=T11 {"nano-position_X_um"=0.0, "nano-position_Y_um"=0.0, "nano-position Z_um"=0.0} ("input_xyz"), "nano-position_X_um"=w496, "nano-position_Y_um"=w495, "nano-position Z_um"=w493) -> (w494:T11)
        n401 = flat-sequence {
          tunnel: path "C:/SpinCore/SpinAPI/lib/spinapi64.dll" ("path in") -> [w503]
          tunnel: [w502] -> w500
          tunnel: [w501] -> w499
          tunnel: w500 -> [_]
          tunnel: w499 -> [_]
          tunnel: w494 -> [w505]
          frame #0 {
            n402 = call "pb-stop.vi"("path in"=w503) -> ("error out"=w501:errorcluster, "path out"=w502:path)  [unwired: 9 in]
            n403 = Wait (ms)(milliseconds to wait=u32 100) -> ()  [unwired: 1 out]
          }
          frame #1 {
            n404 = call "gui_T2.vi"("input_xyz"=w505) -> ()  [unwired: 11 in]
            n405 = property on="laser_on-off" class="Bool (strict)"("Value"=FALSE ("laser_on-off")) -> ()  [unwired: 2 in, 2 out]
          }
        }
      }
      frame "doRecenter" {
        n406 = while {
          stop <- "continious_recenter" continue-if-true
          n407 = property on="scan_image" class="IntGraph (strict)"() -> ("Cursor.Cursor X"=w521:dbl, "Cursor.Cursor Y"=w520:dbl)  [unwired: 2 in, 2 out]
          n408 = property on="focus_z" class="DigNum (strict)"() -> ("Value"=w519:dbl)  [unwired: 2 in, 2 out]
          n409 = Bundle("Cursor.Cursor X"=w521, "Cursor.Cursor Y"=w520, "Value"=w519) -> (w518:T38)  [unwired: 1 in]
          n410 = call "center_particle.vi"("input_xyz"=w518, "parameters_xy-scan"="parameters_xy-scan", "parameters_z-scan"="parameters_z-scan") -> ("output_xyz"=w515:T11)  [unwired: 11 in, 1 out]
          n411 = Unbundle By Name(w515) -> ("nano-position_X_um"=w513:sgl, "nano-position_Y_um"=w512:sgl, "nano-position Z_um"=w514:sgl)
          n412 = property on="scan_image" class="IntGraph (strict)"("Cursor.Cursor X"=w513, "Cursor.Cursor Y"=w512) -> ()  [unwired: 2 in, 2 out]
          n413 = property on="focus_z" class="DigNum (strict)"("Value"=w514) -> ()  [unwired: 2 in, 2 out]
        }
      }
    }
  }
  n414 = Unregister For Events(event registration refnum=w21) -> (error out=w20:errorcluster)  [unwired: 1 in]
  n415 = Destroy User Event(user event=w15, error in=w20) -> ()  [unwired: 1 out]
  n416 = Release Queue(queue=w19) -> ()  [unwired: 2 in, 3 out]
  n417 = call <instrlib>:"PM100D Close.vi"("error in (no error)"=w11, "instrument handle"=w10) -> ()  [unwired: 9 in, 1 out]
